vi "COD主界面（列队使用）.vi"() -> (8 "多列列表框":i32(listbox))   [LabVIEW 2016, in "斯坦道CODMn.lvlib"]
uses:
  <vilib>/Plasmionique/MB Master/MB_Master_Serial/MB_Master_Serial.lvclass
  C:/Program Files (x86)/National Instruments/LabVIEW 2016/vi.lib/Plasmionique/MB Master/MB_Master/MB_Master.lvclass
  <vilib>/Analysis/6fits.llb/Curve Fitting Criteria.ctl
  <vilib>/Utility/miscctls.llb/LVPointTypeDef.ctl
  <vilib>/Utility/config.llb/Read Key (Boolean).vi
  <vilib>/Utility/config.llb/Read Key (I32).vi
  <vilib>/Utility/config.llb/Read Key (Double).vi
  <vilib>/Utility/config.llb/Write Key (Double).vi
  <vilib>/Utility/config.llb/Write Key (Boolean).vi
  <vilib>/Utility/config.llb/Write Key (I32).vi
  <vilib>/Plasmionique/MB Master/MB Master.lvlib
  <vilib>/ptbypt/NI_PtbyPt.lvlib
  PLC/PLC.lvlib
  <vilib>/Utility/config.llb/NI_LVConfig.lvlib
  <vilib>/Analysis/NI_AALPro.lvlib
panel:
  out "空白测试标记":bool
  out "跨度核查标记":bool
  out "启动选择 2":u16(ring) items=["水样测试", "标样核查", "零点核查", "跨度核查", "空白测试", "加标回收", "平行样", "校零", "校标"]
  in  "量程选择":enum16{"低量程", "高量程"}(ring)
  out "MB_Serial session":refnum<class "MB_Master_Serial.lvclass">
  in  "手动控制":bool
  in  "选用水样":enum16{"葡萄糖", "草酸钠"}(ring)
  in  "方程系数":cluster{"X^2":dbl, "X":dbl, "b":dbl} {"X^2" format="%#.4g"; "b" format="%#.4g"; "X" format="%#.4g"}
  out "XY图 2":cluster{"X Values":dbl[], "Y Values":dbl[]}[](graph)
  out "多项式系数1":dbl[](array[numeric]) caption="多项式系数"
  out "多项式系数2":dbl[](array[numeric]) caption="多项式系数"
  out "XY图":cluster{"X Values":dbl[], "Y Values":dbl[]}[](graph)
  in  "模型":enum32{"线性", "多项式"}(ring)
  out "启动时间":timestamp format="%<%Y/%m/%d %H:%M:%S>T"
  in  "自动切换量程":bool=TRUE
  in  "24H周期设置":bool[](xcontrol)
  in  "关闭 2":bool
  in  "周期设置":bool
  out "文本.文本":string
  out "r^2":dbl format="%.4g"
  out "r^2":dbl format="%.8g"
  out "高量程拟合方程":string
  out "拟合公式":string
  out "b 2":dbl format="%#.4g"
  out "K 2":dbl format="%#.4g"
  out "b":dbl format="%#.4g"
  out "K":dbl format="%#.4f"
  out "当前校准":i32
  in  "启用3":bool
  in  "启用2":bool
  in  "启用1":bool
  in  "启用6":bool
  in  "启用5":bool
  in  "校准6":bool
  in  "校准5":bool
  in  "校准4":bool
  in  "启用4":bool
  in  "泵滴定数6":dbl
  in  "泵滴定数5":dbl
  in  "泵滴定数4":dbl
  in  "浓度6":dbl
  in  "浓度5":dbl
  in  "浓度4":dbl
  in  "校准3":bool
  in  "校准2":bool
  in  "校准1":bool
  in  "泵滴定数3":dbl
  in  "泵滴定数2":dbl
  in  "泵滴定数1":dbl
  in  "浓度3":dbl
  in  "浓度2":dbl
  in  "浓度1":dbl
  in  "写入":bool
  out "测量模式数字":i32
  out "零点核查标记":bool
  out "排液故障":bool
  out "进水样超量程":bool
  out "标样核查标记":bool
  out "平行样测量":bool
  out "加标回收测量":bool
  out "质控样测量":bool
  out "待机":bool
  out "校标错误":bool
  out "校零错误":bool
  out "测量错误":bool
  out "草酸钠报警":bool
  out "高锰酸钾报警":bool
  out "加热故障":bool
  out "温控器故障":bool
  out "ORP故障":bool
  out "排液标记":bool
  out "故障标记":bool
  out "校标标记":bool
  out "校零标记":bool
  out "通讯状态":bool
  out "水样测量":bool
  out "读取KB值":bool
  in  "读取":bool
  in  "返回":bool
  in  "校准配置":bool
  in  "修正系数 2":dbl
  in  "浓度 2":dbl
  in  "温度":dbl
  in  "恒温时间":dbl
  in  "基本量程":enum16{"10mL", "20mL"}(ring)
  in  "水样":dbl
  in  "蒸馏水":dbl
  in  "标液":dbl
  in  "质控样":dbl
  in  "加标回收":dbl
  in  "草酸钠":dbl
  in  "高锰酸钾":dbl
  in  "硫酸":dbl
  in  "零点泵计量数 2":dbl
  in  "标度泵计量数 2":dbl
  out "标度滴定值":dbl
  out "零点滴定值":dbl
  in  "保存":bool
  in  "关闭":bool
  out "测量数据区":T1 {"单位" items=["ug/L", "mg/L", "ppm", "mg/m3", "cm", "ppb", "ug/m3", "%", "nmol/mol", "umol/mol", "MPN/L", "MPN/100ml", "ng/m3", "NTU", "无量纲", "ms/cm", "us/cm", "℃", "mV", "万个/L"]}
  out "仪器时间":timestamp format="%<%Y/%m/%d %H:%M:%S>T"
  out "秒":u16
  out "分":u16
  out "COD浓度（mg/L)":dbl format="%.2g"
  out "进样管":dbl
  out "高锰酸钾":dbl
  out "草酸钠":dbl
  out "硫酸":dbl
  out "ORP显示":dbl
  out "温度":dbl
  out "加热":bool
  out "搅拌":bool
  out "进硫酸":bool
  out "进加标回收样":bool
  out "进质控样":bool
  out "进标液":bool
  out "进蒸馏水":bool
  out "进水样":bool
  out "进草酸钠":bool
  out "进高锰酸钾":bool
  in  "定时启动":bool
  in  "启动":bool
  in  "故障清除":bool
  in  "参数配置":bool
  in  "停止":bool
  in  "单步启动":bool
  out "定时时间":dbl
  out "系统时间":timestamp
  in  "时间校准":bool
  in  "枚举":enum16{"读取数据", "写入数据", "读取写入DATABASE", "读取参数"}(ring)
  in  "data in":T2
  out "数值":i32
  out "报警簇":T3
  out "读取参数":u16[](array[numeric])
  out "循环次数":i32
  out "DATABASE":u16[](array[numeric])
  out "Registers":u16[](array[numeric])
  in  "Slave ID":u8=1
  in  "Serial Config":T4={"baud rate (bps)"=115200, "stop bits"=10, "parity"=0, "flow control"=0, "timeout"=1000, "retries"=1} {"stop bits" items=["1.0"=10, "1.5"=15, "2.0"=20]; "flow control" items=["None", "XON/XOFF", "RTS/CTS", "XON/XOFF & RTS/CTS", "DTR/DSR", "XON/XOFF & DTR/DSR"]; "parity" items=["None", "Odd", "Even", "Mark", "Space"]}
  out "table 输入":string
  out "columns":string[](array[string])
  out "data":T5
  in  "温度 2":dbl
  in  "浓度":dbl
  in  "修正系数":dbl
  in  "标样浓度 2":dbl
  out "模式（受控）":u16
  in  "VISA resource name":refnum<visa-resource-name>="COM4" caption="VISA资源名称"
  # "测量时间："
  # "水样~加标回收"
  # "mV"
  # "℃"
  # "注：遇到加热故障和排液故障时仪器不能正常启动，\n必须排查故障并点击报警清除按钮方可运行。"
  # "mg/L"
  # "校零校标结果"
  # "基本参数设置"
  # "泵计量参数设置"
  # "校零结果："
  # "校零滴定值："
  # "加热恒温温度（℃）："
  # "水样："
  # "高锰酸钾："
  # "校标结果："
  # "标度滴定值："
  # "零点泵计量值："
  # "恒温时间（分钟）："
  # "蒸馏水："
  # "草酸钠："
  # "标度泵计量值："
  # "标准液浓度（mg/L）："
  # "标液："
  # "标样浓度："
  # "硫酸："
  # "修正系数："
  # "质控样："
  # "基本量程（20mL可选）："
  # "加标回收样："
  # "是否启用"
  # "泵滴定数"
  # "浓度"
  # "辅\n助\n计\n算\n区"
  # "高量程校准"
  # "泵滴定数"
  # "是否启用"
  # "浓度"
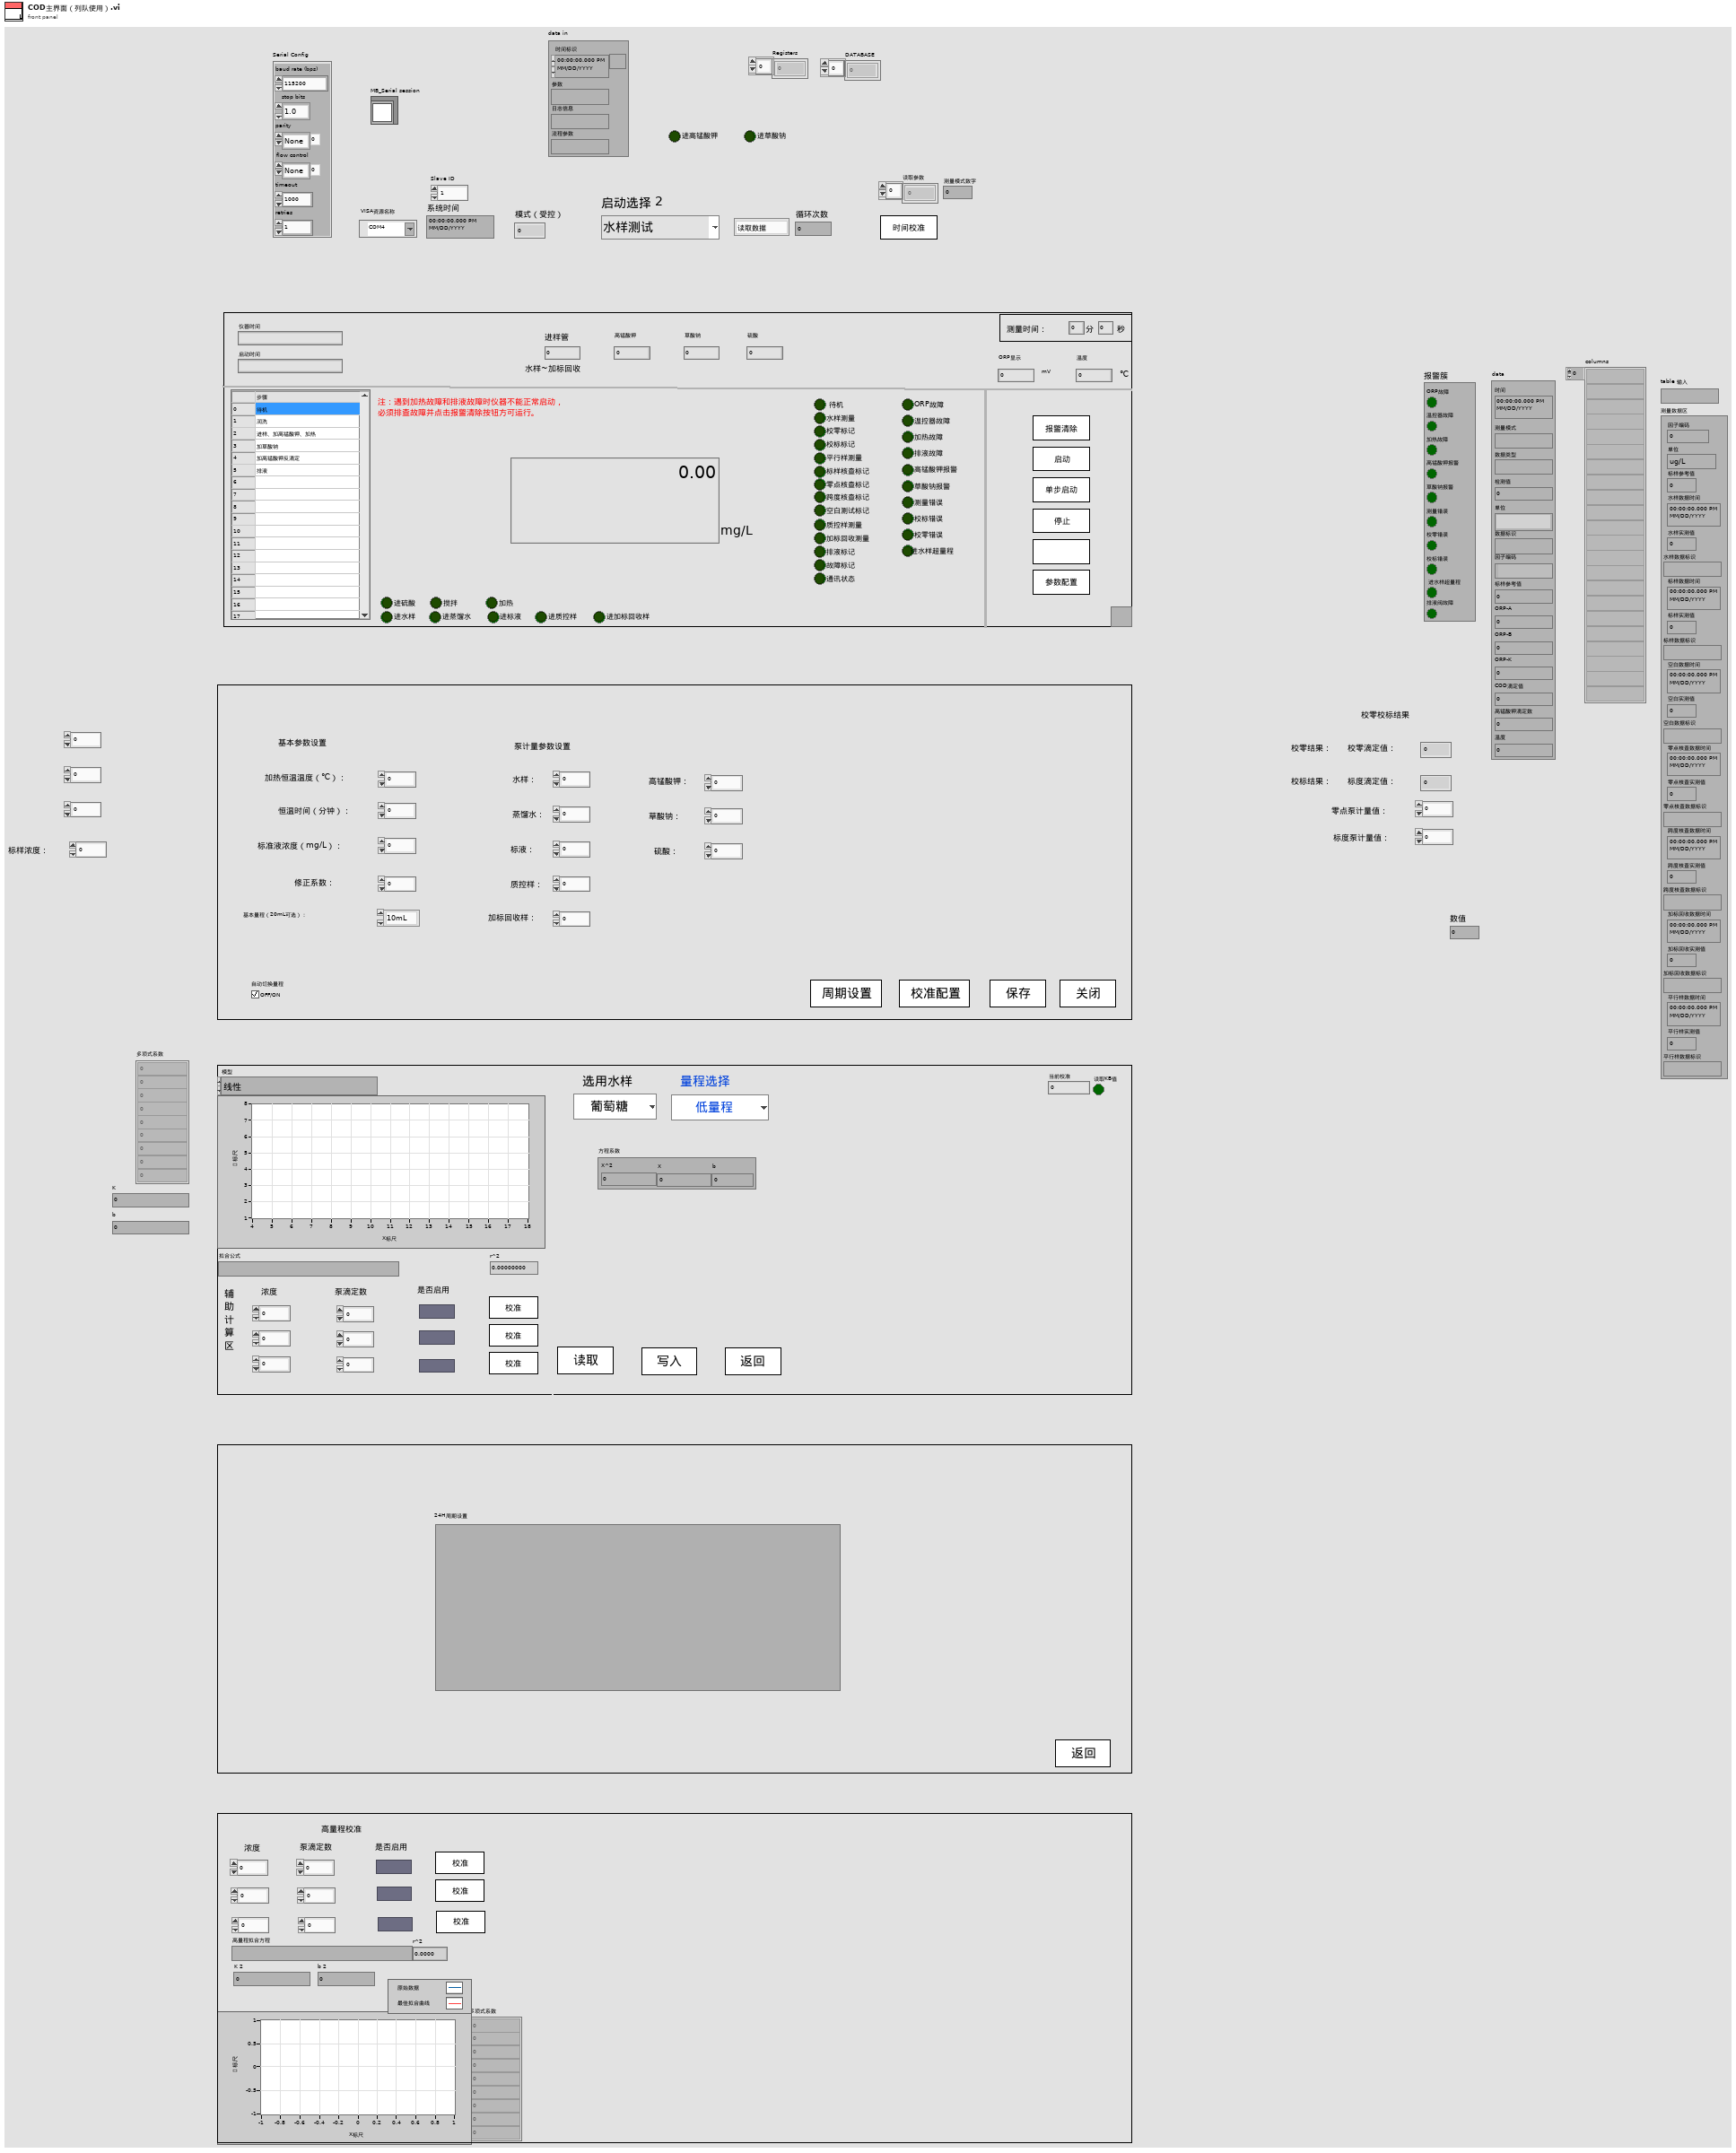
[diagram p1: front panel]
types:
  T1 = cluster{"因子编码":u32, "单位":u16, "标样参考值":sgl, "水样数据时间":timestamp, "水样实测值":sgl, "水样数据标识":string, "标样数据时间":timestamp, "标样实测值":sgl, "标样数据标识":string, "空白数据时间":timestamp, "空白实测值":sgl, "空白数据标识":string, "零点核查数据时间":timestamp, "零点核查实测值":sgl, "零点核查数据标识":string, "跨度核查数据时间":timestamp, "跨度核查实测值":sgl, "跨度核查数据标识":string, "加标回收数据时间":timestamp, "加标回收实测值":sgl, "加标回收数据标识":string, "平行样数据时间":timestamp, "平行样实测值":sgl, "平行样数据标识":string}
  T2 = cluster{"时间标识":timestamp, "参数":string, "日志信息":string, "流程参数":string}
  T3 = cluster{"ORP故障":bool, "温控器故障":bool, "加热故障":bool, "高锰酸钾报警":bool, "草酸钠报警":bool, "测量错误":bool, "校零错误":bool, "校标错误":bool, " 进水样超量程":bool, "排液阀故障":bool}
  T4 = cluster{"baud rate (bps)":u32, "stop bits":u16, "parity":u16, "flow control":u16, "timeout":u32, "retries":i32}
  T5 = cluster{"时间":timestamp, "测量模式":string, "数据类型":string, "检测值":sgl, "单位":string, "数据标识":string, "因子编码":string, "标样参考值":sgl, "ORP-A":sgl, "ORP-B":sgl, "ORP-K":sgl, "COD滴定值":sgl, "高锰酸钾滴定数":sgl, "温度":sgl}
  T6 = cluster{"starting address":u16, "number of holding registers":u16}
  T7 = cluster{"测量模式":enum16{"水样测量", "标样核查", "零点核查", "跨度核查", "空白测试", "加标回收", "平行样", "校零", "校标"}}
  T8 = typedef "LVDateTimeRec.ctl" = cluster{"秒数的小数部分":dbl, "秒":i32, "分":i32, "时":i32, "日":i32, "月":i32, "年":i32, "天数（周）":i32, "天数（年）":i32, "DST":i32}
  T9 = typedef "LVPointTypeDef.ctl" = cluster{"Horizontal":i16, "Vertical":i16}
  T10 = typedef "NI_LVConfig.lvlib/Config Data RefNum.ctl" = refnum<k1>
  T11 = cluster{"时间标识":timestamp, "设备":string, "日志信息":string}
  T12 = typedef "NI_AALPro.lvlib/Curve Fitting Criteria.ctl" = u16
  T13 = cluster{"时间标识":timestamp, "设备":string, "日志信息":string, "流程参数":string}
  T14 = cluster{"数组 2[0]":sgl, "数组 2[1]":sgl, "数组 2[2]":sgl, "数组 2[3]":sgl, "数组 2[4]":sgl, "数组 2[5]":sgl}
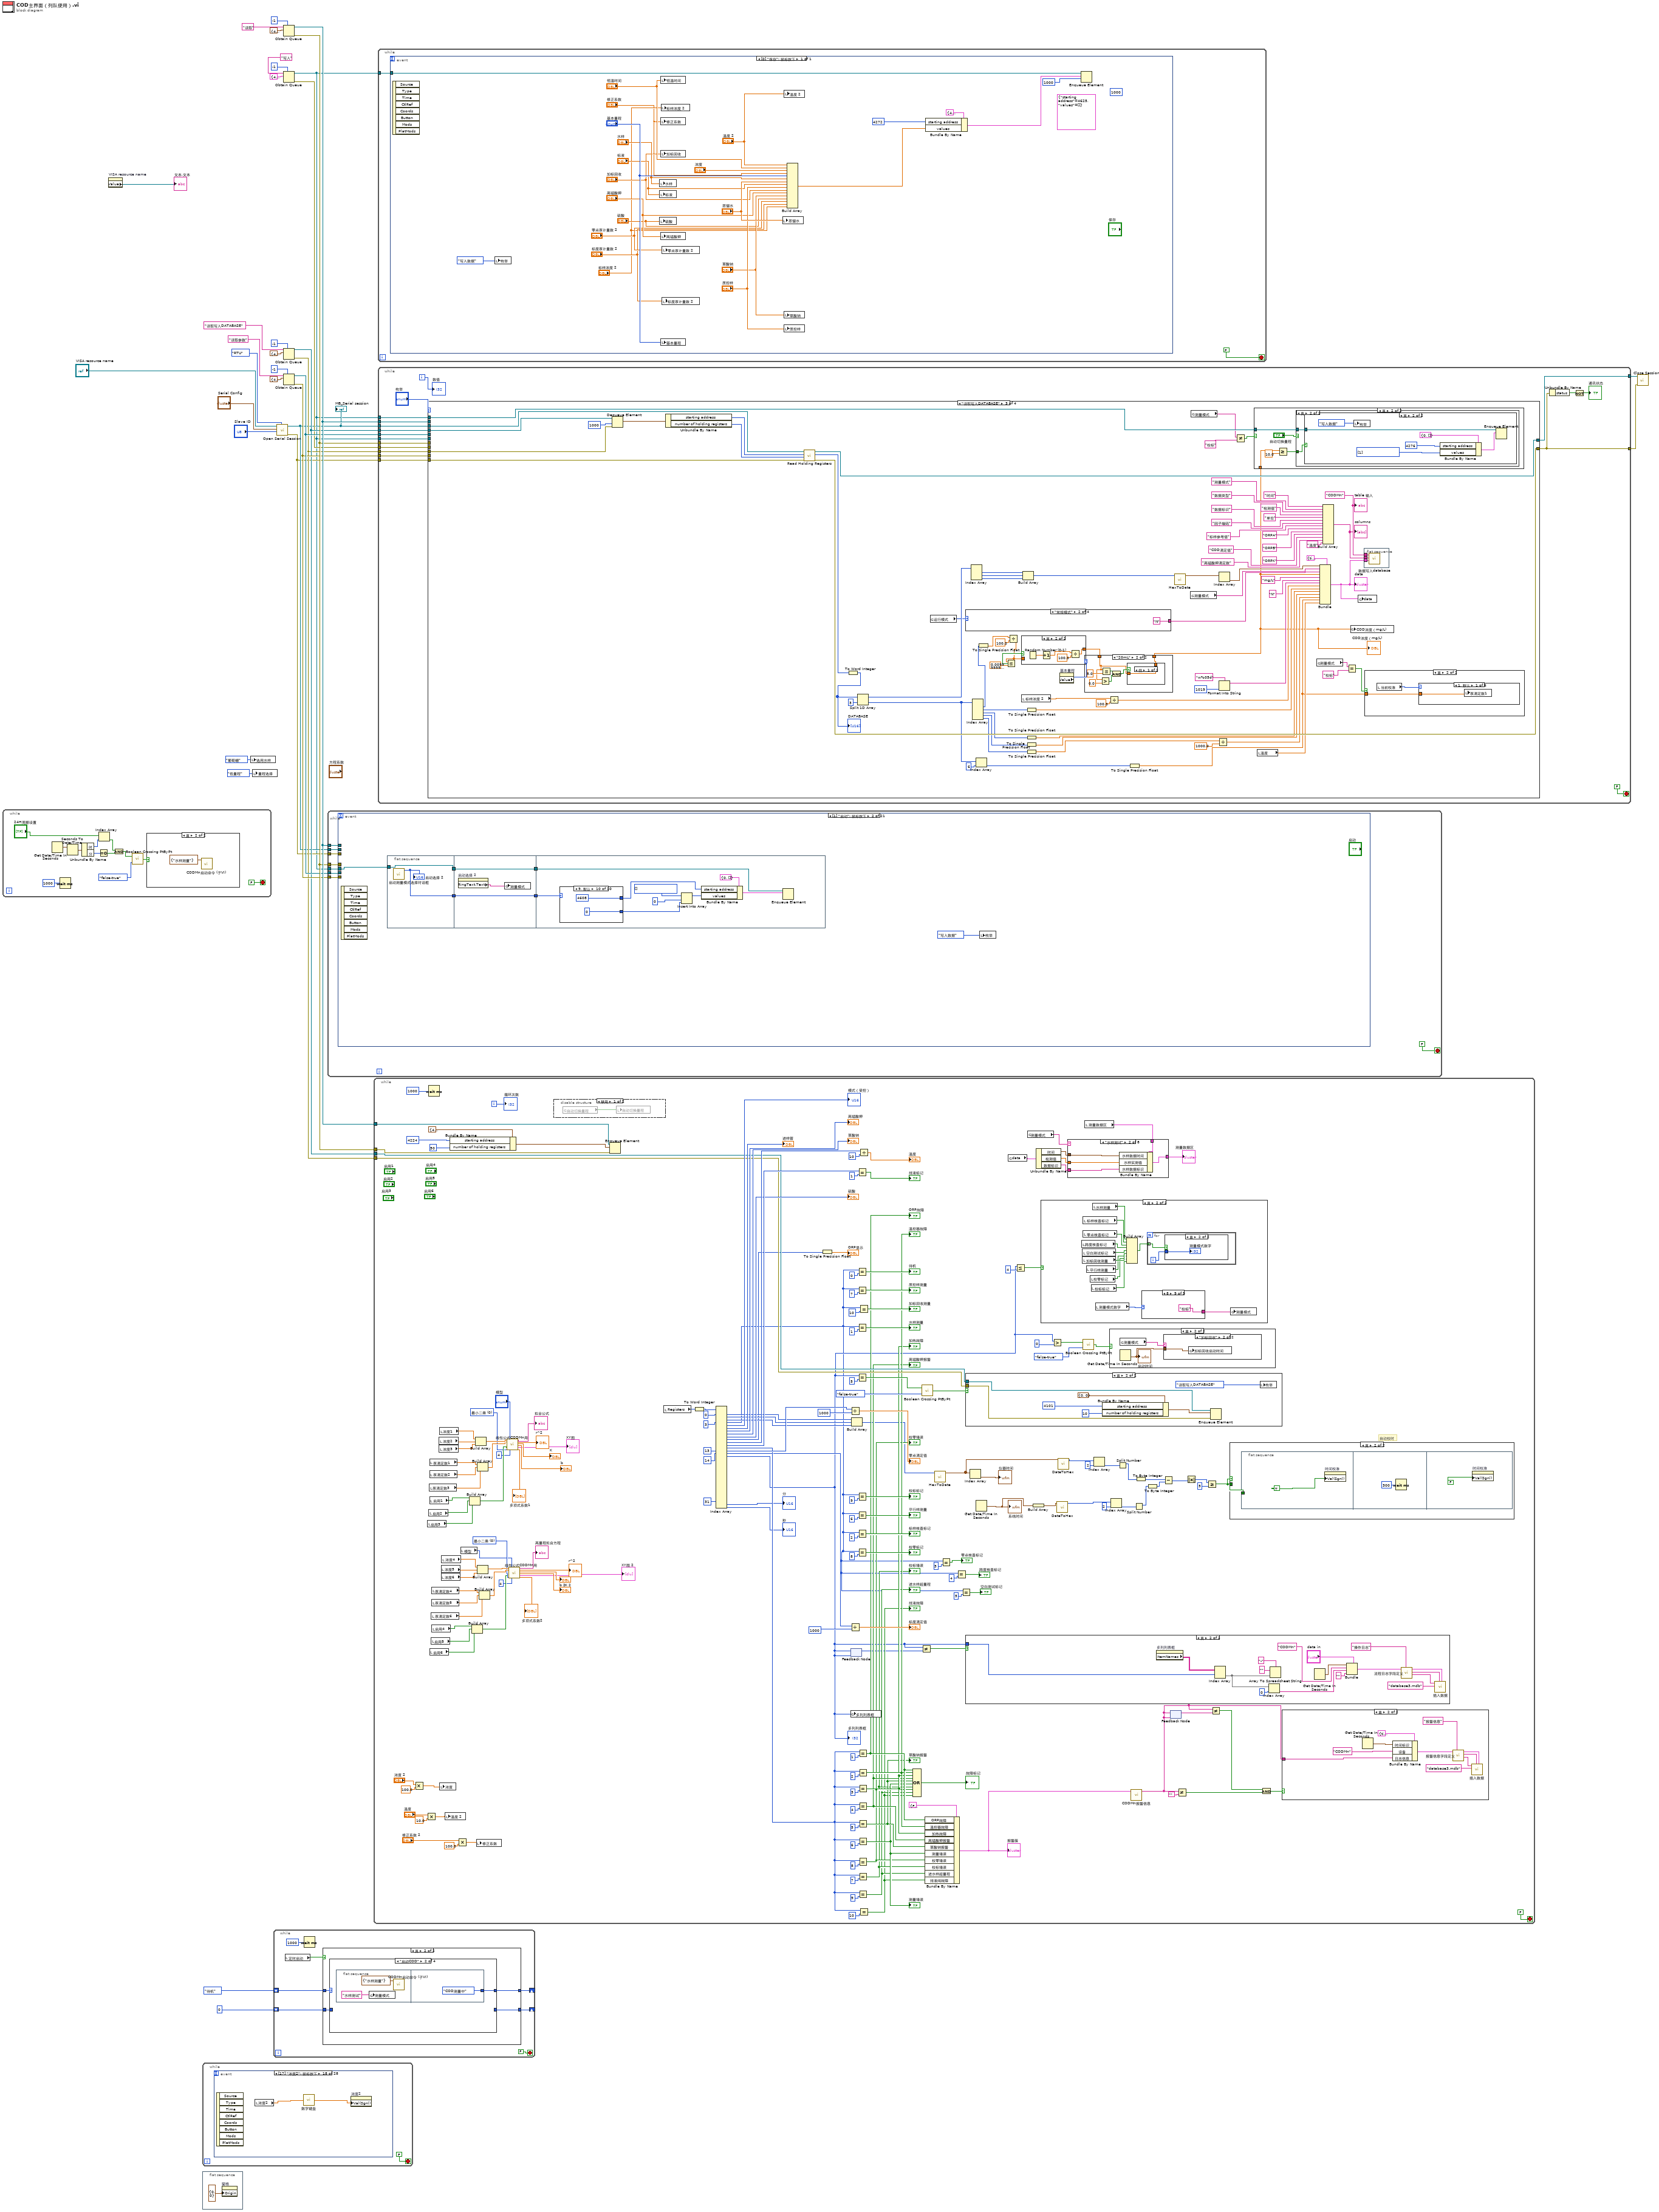
[diagram p0: block diagram]
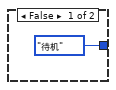
[diagram p3: hidden frame]
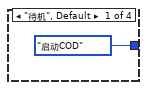
[diagram p4: hidden frame]
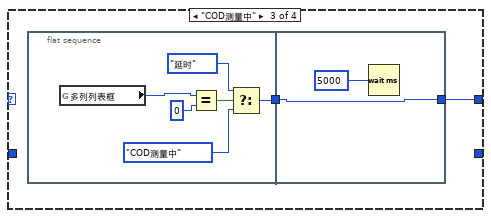
[diagram p5: hidden frame]
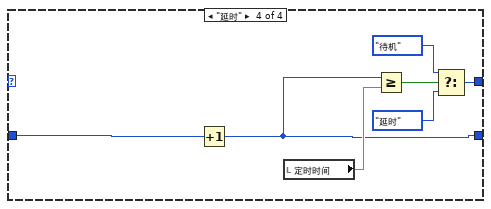
[diagram p6: hidden frame]
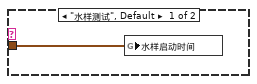
[diagram p9: hidden frame]
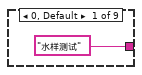
[diagram p11: hidden frame]
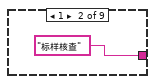
[diagram p12: hidden frame]
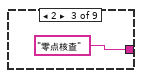
[diagram p13: hidden frame]
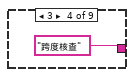
[diagram p14: hidden frame]
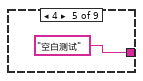
[diagram p15: hidden frame]
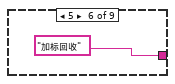
[diagram p16: hidden frame]
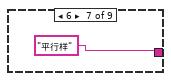
[diagram p17: hidden frame]
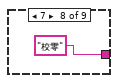
[diagram p18: hidden frame]
diagram:
  n1 = while {
    stop <- FALSE stop-if-true
    n2 = Get Date/Time In Seconds() -> (seconds since 1Jan1904=w45:timestamp)
    n3 = Wait (ms)(milliseconds to wait=u32 1000 ("等待时间（毫秒）")) -> ()  [unwired: 1 out]
    n4 = Seconds To Date/Time(time stamp (now)=w45) -> (date time rec=w44:T8)  [unwired: 1 in]
    n5 = Unbundle By Name(w44) -> ("时"=w41:i32, "分"=w43:i32)
    n6 = Equal To 0?(x=w43) -> (x = 0?=w42:bool)
    n7 = Index Array(array="24H周期设置", index=w41) -> (element=w40:bool)
    n8 = And(x=w40, y=w42) -> (x .and. y?=w38:bool)
    n9 = call <vilib>:"Boolean Crossing PtByPt.vi"("direction"=enum16{"either", "false-true", "true-false"}."false-true", "input"=w38) -> ("crossing"=w37:bool)  [unwired: 1 in]
    n10 = case shown="真" w37 {
      frame False {
      }
      frame True {
        n11 = call "CODMn启动命令 (子VI).vi"("启动测量模式"=T7 {"测量模式"=enum."水样测量"}) -> ()  [unwired: 11 in]
      }
    }
  }
  n12 = property on="VISA resource name" class="VISAName"() -> ("Value"=→"文本.文本":refnum<visa-resource-name>)  [unwired: 2 in, 2 out]
  n13 = while {
    stop <- FALSE stop-if-true
    n14 = event shown="[17] \"浓度2\": 鼠标按下" {
      selector: _ -> [_ _ _ _ _ _ _ _ _ _ _ _ _ _ _ _ _ _ _ _ _ _ _ _ _ _ _ _]
      dyn-events: _ -> [_ _ _ _ _ _ _ _ _ _ _ _ _ _ _ _ _ _ _ _ _ _ _ _ _ _ _ _]
      timeout: _ -> [_ _ _ _ _ _ _ _ _ _ _ _ _ _ _ _ _ _ _ _ _ _ _ _ _ _ _ _]
      event Timeout {
        n15 = event-data() -> ()  [unwired: 1 in, 3 out]
      }
      event "温度": Mouse Down {
        n16 = event-data() -> ()  [unwired: 1 in, 8 out]
        n17 = local read "温度"() -> (w49:dbl)
        n18 = call "数字键盘.vi"("OldNumber"=w49) -> ("NewNumber"=w48:sgl)
        n19 = local write "温度"(w48) -> ()
      }
      event "恒温时间": Mouse Down {
        n20 = event-data() -> ()  [unwired: 1 in, 8 out]
        n21 = local read "恒温时间"() -> (w50:dbl)
        n22 = call "数字键盘.vi"("OldNumber"=w50) -> ("NewNumber"=w51:sgl)
        n23 = local write "恒温时间"(w51) -> ()
      }
      event "浓度 2": Mouse Down {
        n24 = event-data() -> ()  [unwired: 1 in, 8 out]
        n25 = local read "浓度 2"() -> (w53:dbl)
        n26 = call "数字键盘.vi"("OldNumber"=w53) -> ("NewNumber"=w52:sgl)
        n27 = local write "浓度 2"(w52) -> ()
      }
      event "修正系数 2": Mouse Down {
        n28 = event-data() -> ()  [unwired: 1 in, 8 out]
        n29 = local read "修正系数 2"() -> (w54:dbl)
        n30 = call "数字键盘.vi"("OldNumber"=w54) -> ("NewNumber"=w55:sgl)
        n31 = local write "修正系数 2"(w55) -> ()
      }
      event "水样": Mouse Down {
        n32 = event-data() -> ()  [unwired: 1 in, 8 out]
        n33 = local read "水样"() -> (w56:dbl)
        n34 = call "数字键盘.vi"("OldNumber"=w56) -> ("NewNumber"=w57:sgl)
        n35 = local write "水样"(w57) -> ()
      }
      event "蒸馏水": Mouse Down {
        n36 = event-data() -> ()  [unwired: 1 in, 8 out]
        n37 = local read "蒸馏水"() -> (w58:dbl)
        n38 = call "数字键盘.vi"("OldNumber"=w58) -> ("NewNumber"=w59:sgl)
        n39 = local write "蒸馏水"(w59) -> ()
      }
      event "标液": Mouse Down {
        n40 = event-data() -> ()  [unwired: 1 in, 8 out]
        n41 = local read "标液"() -> (w60:dbl)
        n42 = call "数字键盘.vi"("OldNumber"=w60) -> ("NewNumber"=w61:sgl)
        n43 = local write "标液"(w61) -> ()
      }
      event "质控样": Mouse Down {
        n44 = event-data() -> ()  [unwired: 1 in, 8 out]
        n45 = local read "质控样"() -> (w62:dbl)
        n46 = call "数字键盘.vi"("OldNumber"=w62) -> ("NewNumber"=w63:sgl)
        n47 = local write "质控样"(w63) -> ()
      }
      event "加标回收": Mouse Down {
        n48 = event-data() -> ()  [unwired: 1 in, 8 out]
        n49 = local read "加标回收"() -> (w64:dbl)
        n50 = call "数字键盘.vi"("OldNumber"=w64) -> ("NewNumber"=w65:sgl)
        n51 = local write "加标回收"(w65) -> ()
      }
      event "草酸钠": Mouse Down {
        n52 = event-data() -> ()  [unwired: 1 in, 8 out]
        n53 = local read "草酸钠"() -> (w66:dbl)
        n54 = call "数字键盘.vi"("OldNumber"=w66) -> ("NewNumber"=w67:sgl)
        n55 = local write "草酸钠"(w67) -> ()
      }
      event "高锰酸钾": Mouse Down {
        n56 = event-data() -> ()  [unwired: 1 in, 8 out]
        n57 = local read "高锰酸钾"() -> (w68:dbl)
        n58 = call "数字键盘.vi"("OldNumber"=w68) -> ("NewNumber"=w69:sgl)
        n59 = local write "高锰酸钾"(w69) -> ()
      }
      event "硫酸": Mouse Down {
        n60 = event-data() -> ()  [unwired: 1 in, 8 out]
        n61 = local read "硫酸"() -> (w70:dbl)
        n62 = call "数字键盘.vi"("OldNumber"=w70) -> ("NewNumber"=w71:sgl)
        n63 = local write "硫酸"(w71) -> ()
      }
      event "零点泵计量数 2": Mouse Down {
        n64 = event-data() -> ()  [unwired: 1 in, 8 out]
        n65 = local read "零点泵计量数 2"() -> (w72:dbl)
        n66 = call "数字键盘.vi"("OldNumber"=w72) -> ("NewNumber"=w73:sgl)
        n67 = local write "零点泵计量数 2"(w73) -> ()
      }
      event "标度泵计量数 2": Mouse Down {
        n68 = event-data() -> ()  [unwired: 1 in, 8 out]
        n69 = local read "标度泵计量数 2"() -> (w74:dbl)
        n70 = call "数字键盘.vi"("OldNumber"=w74) -> ("NewNumber"=w75:sgl)
        n71 = local write "标度泵计量数 2"(w75) -> ()
      }
      event "标样浓度 2": Mouse Down {
        n72 = event-data() -> ()  [unwired: 1 in, 8 out]
        n73 = local read "标样浓度 2"() -> (w76:dbl)
        n74 = call "数字键盘.vi"("OldNumber"=w76) -> ("NewNumber"=w77:sgl)
        n75 = local write "标样浓度 2"(w77) -> ()
      }
      event "浓度1": Mouse Down {
        n76 = event-data() -> ()  [unwired: 1 in, 8 out]
        n77 = local read "浓度1"() -> (w79:dbl)
        n78 = call "数字键盘.vi"("OldNumber"=w79) -> ("NewNumber"=w78:sgl)
        n79 = property on="浓度1" class="DigNum (严格)"("Val(Sgnl)"=w78) -> ()  [unwired: 2 in, 2 out]
      }
      event "浓度2": Mouse Down {
        n80 = event-data() -> ()  [unwired: 1 in, 8 out]
        n81 = local read "浓度2"() -> (w81:dbl)
        n82 = call "数字键盘.vi"("OldNumber"=w81) -> ("NewNumber"=w80:sgl)
        n83 = property on="浓度2" class="DigNum (严格)"("Val(Sgnl)"=w80) -> ()  [unwired: 2 in, 2 out]
      }
      event "浓度3": Mouse Down {
        n84 = event-data() -> ()  [unwired: 1 in, 8 out]
        n85 = local read "浓度3"() -> (w83:dbl)
        n86 = call "数字键盘.vi"("OldNumber"=w83) -> ("NewNumber"=w82:sgl)
        n87 = property on="浓度3" class="DigNum (严格)"("Val(Sgnl)"=w82) -> ()  [unwired: 2 in, 2 out]
      }
      event "泵滴定数1": Mouse Down {
        n88 = event-data() -> ()  [unwired: 1 in, 8 out]
        n89 = local read "泵滴定数1"() -> (w85:dbl)
        n90 = call "数字键盘.vi"("OldNumber"=w85) -> ("NewNumber"=w84:sgl)
        n91 = property on="泵滴定数1" class="DigNum (严格)"("Val(Sgnl)"=w84) -> ()  [unwired: 2 in, 2 out]
      }
      event "泵滴定数2": Mouse Down {
        n92 = event-data() -> ()  [unwired: 1 in, 8 out]
        n93 = local read "泵滴定数2"() -> (w87:dbl)
        n94 = call "数字键盘.vi"("OldNumber"=w87) -> ("NewNumber"=w86:sgl)
        n95 = property on="泵滴定数2" class="DigNum (严格)"("Val(Sgnl)"=w86) -> ()  [unwired: 2 in, 2 out]
      }
      event "泵滴定数3": Mouse Down {
        n96 = event-data() -> ()  [unwired: 1 in, 8 out]
        n97 = local read "泵滴定数3"() -> (w89:dbl)
        n98 = call "数字键盘.vi"("OldNumber"=w89) -> ("NewNumber"=w88:sgl)
        n99 = property on="泵滴定数3" class="DigNum (严格)"("Val(Sgnl)"=w88) -> ()  [unwired: 2 in, 2 out]
      }
      event "浓度4": Mouse Down {
        n100 = event-data() -> ()  [unwired: 1 in, 8 out]
        n101 = local read "浓度4"() -> (w91:dbl)
        n102 = call "数字键盘.vi"("OldNumber"=w91) -> ("NewNumber"=w90:sgl)
        n103 = property on="浓度4" class="DigNum (严格)"("Val(Sgnl)"=w90) -> ()  [unwired: 2 in, 2 out]
      }
      event "浓度5": Mouse Down {
        n104 = event-data() -> ()  [unwired: 1 in, 8 out]
        n105 = local read "浓度5"() -> (w93:dbl)
        n106 = call "数字键盘.vi"("OldNumber"=w93) -> ("NewNumber"=w92:sgl)
        n107 = property on="浓度5" class="DigNum (严格)"("Val(Sgnl)"=w92) -> ()  [unwired: 2 in, 2 out]
      }
      event "浓度6": Mouse Down {
        n108 = event-data() -> ()  [unwired: 1 in, 8 out]
        n109 = local read "浓度6"() -> (w95:dbl)
        n110 = call "数字键盘.vi"("OldNumber"=w95) -> ("NewNumber"=w94:sgl)
        n111 = property on="浓度6" class="DigNum (严格)"("Val(Sgnl)"=w94) -> ()  [unwired: 2 in, 2 out]
      }
      event "泵滴定数4": Mouse Down {
        n112 = event-data() -> ()  [unwired: 1 in, 8 out]
        n113 = local read "泵滴定数4"() -> (w97:dbl)
        n114 = call "数字键盘.vi"("OldNumber"=w97) -> ("NewNumber"=w96:sgl)
        n115 = property on="泵滴定数4" class="DigNum (严格)"("Val(Sgnl)"=w96) -> ()  [unwired: 2 in, 2 out]
      }
      event "泵滴定数5": Mouse Down {
        n116 = event-data() -> ()  [unwired: 1 in, 8 out]
        n117 = local read "泵滴定数5"() -> (w99:dbl)
        n118 = call "数字键盘.vi"("OldNumber"=w99) -> ("NewNumber"=w98:sgl)
        n119 = property on="泵滴定数5" class="DigNum (严格)"("Val(Sgnl)"=w98) -> ()  [unwired: 2 in, 2 out]
      }
      event "泵滴定数6": Mouse Down {
        n120 = event-data() -> ()  [unwired: 1 in, 8 out]
        n121 = local read "泵滴定数6"() -> (w101:dbl)
        n122 = call "数字键盘.vi"("OldNumber"=w101) -> ("NewNumber"=w100:sgl)
        n123 = property on="泵滴定数6" class="DigNum (严格)"("Val(Sgnl)"=w100) -> ()  [unwired: 2 in, 2 out]
      }
    }
  }
  n124 = flat-sequence {
    frame #0 {
      n125 = property on="窗格" class="Pane"("Origin"=T9 {"Horizontal"=0, "Vertical"=0} ("原点")) -> ()  [unwired: 2 in, 2 out]
    }
  }
  n126 = local write "选用水样"(enum16{"葡萄糖", "草酸钠"}."葡萄糖" ("选用水样")) -> ()
  n127 = local write "量程选择"(enum16{"低量程", "高量程"}."低量程" ("量程选择")) -> ()
  n128 = while {
    shift-right: [w104] -> _
    shift-left: enum16{"待机", "启动COD", "COD测量中", "延时"}."待机" -> [w106]
    shift-right: [w103] -> _
    shift-left: 0 -> [w105]
    stop <- FALSE stop-if-true
    n129 = local read "定时启动"() -> (w108:bool)
    n130 = Wait (ms)(milliseconds to wait=u32 1000 ("等待时间（毫秒）")) -> ()  [unwired: 1 out]
    n131 = case shown="真" w108 {
      tunnel: w106 -> [_ w114]
      tunnel: w105 -> [_ w113]
      tunnel: [enum16{"待机", "启动COD", "COD测量中", "延时"}."待机" w112] -> w104
      tunnel: [_ w111] -> w103
      frame False {
      }
      frame True {
        n132 = case shown="\"启动COD\"" w114 {
          tunnel: w113 -> [_ _ _ w136]
          tunnel: [enum16{"待机", "启动COD", "COD测量中", "延时"}."启动COD" w116 w121 w130] -> w112
          tunnel: [_ _ _ w133] -> w111
          frame "待机", Default {
          }
          frame "启动COD" {
            n133 = flat-sequence {
              tunnel: [enum16{"待机", "启动COD", "COD测量中", "延时"}."COD测量中"] -> w116
              frame #0 {
                n134 = global write "COD测量模式全局.vi" "测量模式"("水样测试" ("测量模式")) -> ()
                n135 = call "CODMn启动命令 (子VI).vi"("启动测量模式"=T7 {"测量模式"=enum."水样测量"}) -> ()  [unwired: 11 in]
              }
              frame #1 {
              }
            }
          }
          frame "COD测量中" {
            n136 = flat-sequence {
              tunnel: [w122] -> w120
              tunnel: [w129] -> w121
              tunnel: w120 -> [w129]
              frame #0 {
                n137 = global read "运行时序全局变量.vi" "多列列表框"() -> (w127:i32)
                n138 = Equal?(x=w127, y=0) -> (x = y?=w125:bool)
                n139 = Select(t=enum16{"待机", "启动COD", "COD测量中", "延时"}."延时", s=w125, f=enum16{"待机", "启动COD", "COD测量中", "延时"}."COD测量中") -> (s? t:f=w122:enum16{"待机", "启动COD", "COD测量中", "延时"})
              }
              frame #1 {
                n140 = Wait (ms)(milliseconds to wait=u32 5000 ("等待时间（毫秒）")) -> ()  [unwired: 1 out]
              }
            }
          }
          frame "延时" {
            n141 = Increment(x=w136) -> (x+1=w133:i32)
            n142 = local read "定时时间"() -> (w135:dbl)
            n143 = Greater Or Equal?(x=w133, y=w135) -> (x >= y?=w134:bool)
            n144 = Select(t=enum16{"待机", "启动COD", "COD测量中", "延时"}."待机", s=w134, f=enum16{"待机", "启动COD", "COD测量中", "延时"}."延时") -> (s? t:f=w130:enum16{"待机", "启动COD", "COD测量中", "延时"})
          }
        }
      }
    }
  }
  n145 = call <vilib>:"Open Serial Session.vi"("Mode (RTU)"=enum16{"RTU", "ASCII"}."RTU", "Slave ID"="Slave ID", "Serial Config"="Serial Config", "VISA Resource"="VISA resource name") -> ("Error out"=w7:errorcluster, "MB_Serial session"=w8:refnum<class "MB_Master_Serial.lvclass">)  [unwired: 6 in]
  "MB_Serial session" <- w8
  n146 = Obtain Queue(max queue size (-1, unlimited)=-1 ("队列最大值（-1，无限）"), name (unnamed)="读取" ("名称（未命名）"), element data type=T6 {"starting address"=4224, "number of holding registers"=16}) -> (queue out=w23:refnum<queue>, error out=w22:errorcluster)  [unwired: 2 in, 1 out]
  n147 = Obtain Queue(max queue size (-1, unlimited)=-1 ("队列最大值（-1，无限）"), name (unnamed)="写入" ("名称（未命名）"), element data type=cluster{"starting address":u16, "values":u16[]} {"starting address"=4272, "values"=[]}) -> (queue out=w4:refnum<queue>, error out=w9:errorcluster)  [unwired: 2 in, 1 out]
  n148 = Obtain Queue(max queue size (-1, unlimited)=-1 ("队列最大值（-1，无限）"), name (unnamed)="读取写入DATABASE" ("名称（未命名）"), element data type=T6 {"starting address"=4224, "number of holding registers"=16}) -> (queue out=w11:refnum<queue>, error out=w10:errorcluster)  [unwired: 2 in, 1 out]
  n149 = Obtain Queue(max queue size (-1, unlimited)=-1 ("队列最大值（-1，无限）"), name (unnamed)="读取参数" ("名称（未命名）"), element data type=T6 {"starting address"=4224, "number of holding registers"=16}) -> (queue out=w16:refnum<queue>, error out=w15:errorcluster)  [unwired: 2 in, 1 out]
  n150 = while {
    tunnel: w23 -> [w144]
    tunnel: w22 -> [w143]
    tunnel: w4 -> [w142]
    tunnel: w16 -> [w141]
    tunnel: w15 -> [w140]
    tunnel: w8 -> [w138]
    tunnel: w7 -> [w137]
    stop <- FALSE stop-if-true
    n151 = event shown="[1] \"启动\": 鼠标按下" {
      selector: _ -> [_ _ _ _ _ _ _ _ _ _ _ _ _ _ _ _ _ _ _ _ _]
      dyn-events: _ -> [_ _ _ _ _ _ _ _ _ _ _ _ _ _ _ _ _ _ _ _ _]
      timeout: _ -> [_ _ _ _ _ _ _ _ _ _ _ _ _ _ _ _ _ _ _ _ _]
      tunnel: w144 -> [_ _ _ _ _ _ _ _ _ _ _ _ _ _ _ _ _ _ _ _ _]
      tunnel: w143 -> [_ _ _ _ _ _ _ _ _ _ _ _ _ _ _ _ _ _ _ _ _]
      tunnel: w142 -> [w152 w185 w222 _ _ _ _ _ _ _ _ _ w623 w637 _ w645 _ _ _ _ w838]
      tunnel: w141 -> [_ _ _ _ w241 _ _ _ _ _ _ _ _ _ _ _ _ _ _ w830 _]
      tunnel: w140 -> [_ _ _ _ w240 _ _ _ _ _ _ _ _ _ _ _ _ _ _ w829 _]
      tunnel: w138 -> [_ _ _ w228 _ _ _ _ _ _ _ w622 _ _ _ _ _ _ _ _ _]
      tunnel: w137 -> [_ _ _ w227 _ _ _ _ _ _ _ w621 _ _ _ _ _ _ _ _ _]
      event "单步启动": Mouse Down {
        n152 = event-data() -> ()  [unwired: 1 in, 8 out]
        n153 = call "单步启动选择对话框.vi"() -> ("启动选择2"=w145:u16)  [unwired: 10 in, 1 out]
        n154 = case shown="12, 默认" w145 {
          tunnel: [u16 4610 ("address") u16 4610 ("address") u16 4610 ("address") u16 4610 ("address") u16 4610 ("address") u16 4610 ("address") u16 4610 ("address") u16 4610 ("address") u16 4610 ("address") u16 4610 ("address") u16 4610 ("address") u16 4610 ("address") u16 4610 ("address")] -> w151
          tunnel: [u16 1 ("address") u16 2 ("address") u16 3 ("address") u16 4 ("address") u16 5 ("address") u16 6 ("address") u16 7 ("address") u16 8 ("address") u16 9 ("holding register value") u16 10 ("holding register value") u16 11 ("holding register value") u16 12 ("address") u16 0 ("address")] -> w148
          frame 0 {
          }
          frame 1 {
          }
          frame 2 {
          }
          frame 3 {
          }
          frame 4 {
          }
          frame 5 {
          }
          frame 6 {
          }
          frame 7 {
          }
          frame 8 {
          }
          frame 9 {
          }
          frame 10 {
          }
          frame 11 {
          }
          frame 12, Default {
          }
        }
        n155 = local write "枚举"(enum16{"读取数据", "写入数据", "读取写入DATABASE", "读取参数"}."写入数据" ("枚举")) -> ()
        n156 = Insert Into Array(array=u16[] [] ("values"), index=0 ("索引"), new element=w148) -> (w147:u16[])
        n157 = Bundle By Name(cluster=cluster{"starting address":u16, "values":u16[]} {"starting address"=0, "values"=[]}, "starting address"=w151, "values"=w147) -> (w153:cluster{"starting address":u16, "values":u16[]})
        n158 = Enqueue Element(queue=w152, element=w153) -> ()  [unwired: 2 in, 3 out]
      }
      event "启动": Mouse Down {
        n159 = event-data() -> ()  [unwired: 1 in, 8 out]
        n160 = flat-sequence {
          tunnel: w185 -> [w188]
          tunnel: [w188] -> w184
          tunnel: [w187] -> w181
          tunnel: w184 -> [w191]
          tunnel: [w191] -> w183
          tunnel: [w189] -> w182
          tunnel: w181 -> [w189]
          tunnel: w183 -> [w193]
          tunnel: w182 -> [w192]
          frame #0 {
            n161 = call "启动测量模式选择对话框.vi"() -> ("启动选择 2"=w187:u16)  [unwired: 11 in]
            "启动选择 2" <- w187
          }
          frame #1 {
            n162 = property on="启动选择 2" class="Ring (严格)"() -> ("RingText.Text"=w190:string)  [unwired: 2 in, 2 out]
            n163 = global write "COD测量模式全局.vi" "测量模式"(w190) -> ()
          }
          frame #2 {
            n164 = case shown="9, 默认" w192 {
              tunnel: [u16 4608 ("address") u16 4608 ("address") u16 4608 ("address") u16 4608 ("address") u16 4608 ("address") u16 4608 ("address") u16 4608 ("address") u16 4608 ("address") u16 4608 ("address") u16 4608 ("address")] -> w194
              tunnel: [u16 1 ("address") u16 2 ("address") u16 3 ("address") u16 4 ("address") u16 5 ("address") u16 7 ("address") u16 6 ("address") u16 8 ("address") u16 9 ("address") u16 0 ("address")] -> w195
              frame 0 {
              }
              frame 1 {
              }
              frame 2 {
              }
              frame 3 {
              }
              frame 4 {
              }
              frame 5 {
              }
              frame 6 {
              }
              frame 7 {
              }
              frame 8 {
              }
              frame 9, Default {
              }
            }
            n165 = Insert Into Array(array=u16[] [] ("values"), index=0 ("索引"), new element=w195) -> (w200:u16[])
            n166 = Bundle By Name(cluster=cluster{"starting address":u16, "values":u16[]} {"starting address"=0, "values"=[]}, "starting address"=w194, "values"=w200) -> (w197:cluster{"starting address":u16, "values":u16[]})
            n167 = Enqueue Element(queue=w193, element=w197) -> ()  [unwired: 2 in, 3 out]
          }
        }
        n168 = local write "枚举"(enum16{"读取数据", "写入数据", "读取写入DATABASE", "读取参数"}."写入数据" ("枚举")) -> ()
      }
      event "停止": Value Change {
        n169 = event-data() -> ()  [unwired: 1 in, 6 out]
        n170 = local write "枚举"(enum16{"读取数据", "写入数据", "读取写入DATABASE", "读取参数"}."写入数据" ("枚举")) -> ()
        n171 = Bundle By Name(cluster=cluster{"starting address":u16, "values":u16[]} {"starting address"=0, "values"=[]}, "starting address"=u16 4608, "values"=u16[] [11]) -> (w224:cluster{"starting address":u16, "values":u16[]})
        n172 = Enqueue Element(queue=w222, element=w224) -> ()  [unwired: 2 in, 3 out]
      }
      event "手动控制": Value Change {
        n173 = event-data() -> ()  [unwired: 1 in, 6 out]
        n174 = call "CODMn手动控制框.vi"("Error in"=w227, "MB_Serial session"=w228) -> ()  [unwired: 10 in]
      }
      event "参数配置": Value Change {
        n175 = event-data() -> ()  [unwired: 1 in, 6 out]
        n176 = property on="窗格" class="Pane"("Origin"=T9 {"Horizontal"=0, "Vertical"=650} ("原点")) -> ()  [unwired: 2 in, 2 out]
        n177 = Bundle By Name(cluster=T6 {"starting address"=0, "number of holding registers"=0}, "starting address"=u16 4240, "number of holding registers"=u16 16) -> (w248:T6)
        n178 = local write "读取KB值"(FALSE ("读取KB值")) -> ()
        n179 = local write "枚举"(enum16{"读取数据", "写入数据", "读取写入DATABASE", "读取参数"}."读取参数" ("枚举")) -> ()
        n180 = Flush Queue(queue=w241, error in (no error)=w240) -> (queue out=w244:refnum<queue>, error out=w243:errorcluster)  [unwired: 1 out]
        n181 = Enqueue Element(queue=w244, element=w248, error in (no error)=w243) -> ()  [unwired: 1 in, 3 out]
        n182 = call <vilib>:"Application Directory.vi"() -> ("Application Directory"=w236:path)
        n183 = Build Path(base path=w236, name or relative path="data\\Set.ini" ("名称或相对路径")) -> (appended path=w234:path)
        n184 = call <vilib>:"Open Config Data.vi"("configuration file path"=w234) -> ("error out"=w237:errorcluster, "refnum"=w238:T10)  [unwired: 8 in, 1 out]
        n185 = call-poly <vilib>:"Read Key.vi"("section"="CODMn是否切换量程" ("key"), "error in (no error)"=w237, "key"="自动切换量程", "refnum"=w238) -> ("error out"=w230:errorcluster, "value"=w229:bool, "refnum out"=w231:T10)  [unwired: 4 in, 1 out]
        n186 = local write "自动切换量程"(w229) -> ()
        n187 = call <vilib>:"Close Config Data.vi"("error in (no error)"=w230, "refnum"=w231) -> ()  [unwired: 8 in, 2 out]
      }
      event "校准配置": Value Change {
        n188 = event-data() -> ()  [unwired: 1 in, 6 out]
        n189 = property on="窗格" class="Pane"("Origin"=T9 {"Horizontal"=0, "Vertical"=1300} ("原点")) -> ()  [unwired: 2 in, 2 out]
        n190 = call <vilib>:"Application Directory.vi"() -> ("Application Directory"=w298:path)
        n191 = Build Path(base path=w298, name or relative path="data\\Set.ini" ("名称或相对路径")) -> (appended path=w296:path)
        n192 = call <vilib>:"Open Config Data.vi"("configuration file path"=w296) -> ("error out"=w258:errorcluster, "refnum"=w259:T10)  [unwired: 8 in, 1 out]
        n193 = call-poly <vilib>:"Read Key.vi"("section"="CODMn模型选择" ("key"), "error in (no error)"=w258, "key"="线性和多项式", "refnum"=w259) -> ("error out"=w254:errorcluster, "value"=w257:i32, "refnum out"=w255:T10)  [unwired: 4 in, 1 out]
        n194 = local write "模型"(w257) -> ()
        n195 = call-poly <vilib>:"Read Key.vi"("section"="标线选择", "error in (no error)"=w254, "key"="选用水样", "refnum"=w255) -> ("error out"=w252:errorcluster, "value"=w256:i32, "refnum out"=w253:T10)  [unwired: 4 in, 1 out]
        n196 = local write "选用水样"(w256) -> ()
        n197 = local read "量程选择"() -> (w265:enum16{"低量程", "高量程"})
        n198 = case shown="0, 默认" w256 {
          tunnel: ["葡萄糖标线" ("section") "草酸钠标线" ("section")] -> w264
          frame 0, Default {
          }
          frame 1 {
          }
        }
        n199 = case shown="\"高量程\"" w265 {
          tunnel: ["低量程" "高量程"] -> w263
          frame "低量程", Default {
          }
          frame "高量程" {
          }
        }
        n200 = Concatenate Strings(w264, w263) -> (w262:string)
        n201 = call-poly <vilib>:"Read Key.vi"("section"=w262, "error in (no error)"=w252, "key"="浓度1", "refnum"=w253) -> ("error out"=w302:errorcluster, "value"=w300:dbl, "refnum out"=w301:T10)  [unwired: 4 in, 1 out]
        n202 = local write "浓度1"(w300) -> ()
        n203 = call-poly <vilib>:"Read Key.vi"("section"=w262, "error in (no error)"=w302, "key"="浓度2", "refnum"=w301) -> ("error out"=w316:errorcluster, "value"=w303:dbl, "refnum out"=w315:T10)  [unwired: 4 in, 1 out]
        n204 = local write "浓度2"(w303) -> ()
        n205 = call-poly <vilib>:"Read Key.vi"("section"=w262, "error in (no error)"=w316, "key"="浓度3", "refnum"=w315) -> ("error out"=w317:errorcluster, "value"=w305:dbl, "refnum out"=w314:T10)  [unwired: 4 in, 1 out]
        n206 = local write "浓度3"(w305) -> ()
        n207 = call-poly <vilib>:"Read Key.vi"("section"=w262, "error in (no error)"=w317, "key"="泵滴定数1", "refnum"=w314) -> ("error out"=w318:errorcluster, "value"=w307:dbl, "refnum out"=w313:T10)  [unwired: 4 in, 1 out]
        n208 = local write "泵滴定数1"(w307) -> ()
        n209 = call-poly <vilib>:"Read Key.vi"("section"=w262, "error in (no error)"=w318, "key"="泵滴定数2", "refnum"=w313) -> ("error out"=w312:errorcluster, "value"=w310:dbl, "refnum out"=w319:T10)  [unwired: 4 in, 1 out]
        n210 = local write "泵滴定数2"(w310) -> ()
        n211 = call-poly <vilib>:"Read Key.vi"("section"=w262, "error in (no error)"=w312, "key"="泵滴定数3", "refnum"=w319) -> ("error out"=w327:errorcluster, "value"=w326:dbl, "refnum out"=w320:T10)  [unwired: 4 in, 1 out]
        n212 = local write "泵滴定数3"(w326) -> ()
        n213 = call-poly <vilib>:"Read Key.vi"("section"=w262, "error in (no error)"=w327, "key"="浓度4", "refnum"=w320) -> ("error out"=w328:errorcluster, "value"=w334:dbl, "refnum out"=w321:T10)  [unwired: 4 in, 1 out]
        n214 = local write "浓度4"(w334) -> ()
        n215 = call-poly <vilib>:"Read Key.vi"("section"=w262, "error in (no error)"=w328, "key"="浓度5", "refnum"=w321) -> ("error out"=w329:errorcluster, "value"=w335:dbl, "refnum out"=w322:T10)  [unwired: 4 in, 1 out]
        n216 = local write "浓度5"(w335) -> ()
        n217 = call-poly <vilib>:"Read Key.vi"("section"=w262, "error in (no error)"=w329, "key"="浓度6", "refnum"=w322) -> ("error out"=w330:errorcluster, "value"=w336:dbl, "refnum out"=w323:T10)  [unwired: 4 in, 1 out]
        n218 = local write "浓度6"(w336) -> ()
        n219 = call-poly <vilib>:"Read Key.vi"("section"=w262, "error in (no error)"=w330, "key"="泵滴定数4", "refnum"=w323) -> ("error out"=w331:errorcluster, "value"=w337:dbl, "refnum out"=w324:T10)  [unwired: 4 in, 1 out]
        n220 = local write "泵滴定数4"(w337) -> ()
        n221 = call-poly <vilib>:"Read Key.vi"("section"=w262, "error in (no error)"=w331, "key"="泵滴定数5", "refnum"=w324) -> ("error out"=w332:errorcluster, "value"=w338:dbl, "refnum out"=w325:T10)  [unwired: 4 in, 1 out]
        n222 = local write "泵滴定数5"(w338) -> ()
        n223 = call-poly <vilib>:"Read Key.vi"("section"=w262, "error in (no error)"=w332, "key"="泵滴定数6", "refnum"=w325) -> ("error out"=w292:errorcluster, "value"=w339:dbl, "refnum out"=w295:T10)  [unwired: 4 in, 1 out]
        n224 = local write "泵滴定数6"(w339) -> ()
        n225 = call-poly <vilib>:"Read Key.vi"("section"=w262, "error in (no error)"=w292, "key"="当前选用的校准", "refnum"=w295) -> ("error out"=w290:errorcluster, "value"=w293:i32, "refnum out"=w291:T10)  [unwired: 4 in, 1 out]
        n226 = local write "当前校准"(w293) -> ()
        n227 = call-poly <vilib>:"Read Key.vi"("section"=w262, "error in (no error)"=w290, "key"="启用1", "refnum"=w291) -> ("error out"=w287:errorcluster, "value"=w273:bool, "refnum out"=w288:T10)  [unwired: 4 in, 1 out]
        n228 = local write "启用1"(w273) -> ()
        n229 = call-poly <vilib>:"Read Key.vi"("section"=w262, "error in (no error)"=w287, "key"="启用2", "refnum"=w288) -> ("error out"=w285:errorcluster, "value"=w272:bool, "refnum out"=w286:T10)  [unwired: 4 in, 1 out]
        n230 = local write "启用2"(w272) -> ()
        n231 = call-poly <vilib>:"Read Key.vi"("section"=w262, "error in (no error)"=w285, "key"="启用3", "refnum"=w286) -> ("error out"=w283:errorcluster, "value"=w271:bool, "refnum out"=w284:T10)  [unwired: 4 in, 1 out]
        n232 = local write "启用3"(w271) -> ()
        n233 = call-poly <vilib>:"Read Key.vi"("section"=w262, "error in (no error)"=w283, "key"="启用4", "refnum"=w284) -> ("error out"=w281:errorcluster, "value"=w270:bool, "refnum out"=w282:T10)  [unwired: 4 in, 1 out]
        n234 = local write "启用4"(w270) -> ()
        n235 = call-poly <vilib>:"Read Key.vi"("section"=w262, "error in (no error)"=w281, "key"="启用5", "refnum"=w282) -> ("error out"=w279:errorcluster, "value"=w269:bool, "refnum out"=w280:T10)  [unwired: 4 in, 1 out]
        n236 = local write "启用5"(w269) -> ()
        n237 = call-poly <vilib>:"Read Key.vi"("section"=w262, "error in (no error)"=w279, "key"="启用6", "refnum"=w280) -> ("error out"=w250:errorcluster, "value"=w268:bool, "refnum out"=w251:T10)  [unwired: 4 in, 1 out]
        n238 = local write "启用6"(w268) -> ()
        n239 = call <vilib>:"Close Config Data.vi"("error in (no error)"=w250, "refnum"=w251) -> ()  [unwired: 8 in, 2 out]
      }
      event "选用水样": Value Change {
        (unwired) "选用水样" ("key")
        (unwired) "标线选择" ("section")
        n240 = event-data() -> ()  [unwired: 1 in, 6 out]
        n241 = property on="窗格" class="Pane"("Origin"=T9 {"Horizontal"=0, "Vertical"=1300} ("原点")) -> ()  [unwired: 2 in, 2 out]
        n242 = local read "量程选择"() -> (w351:enum16{"低量程", "高量程"})
        n243 = case shown="\"高量程\"" w351 {
          tunnel: ["低量程" "高量程"] -> w352
          frame "低量程", Default {
          }
          frame "高量程" {
          }
        }
        n244 = case shown="\"葡萄糖\", 默认" "选用水样" {
          tunnel: ["葡萄糖标线" ("section") "草酸钠标线" ("section")] -> w353
          frame "葡萄糖", Default {
          }
          frame "草酸钠" {
          }
        }
        n245 = call <vilib>:"Application Directory.vi"() -> ("Application Directory"=w387:path)
        n246 = Build Path(base path=w387, name or relative path="data\\Set.ini" ("名称或相对路径")) -> (appended path=w385:path)
        n247 = call <vilib>:"Open Config Data.vi"("configuration file path"=w385) -> ("error out"=w388:errorcluster, "refnum"=w389:T10)  [unwired: 8 in, 1 out]
        n248 = Concatenate Strings(w353, w352) -> (w350:string)
        n249 = call-poly <vilib>:"Read Key.vi"("section"=w350, "error in (no error)"=w388, "key"="浓度1", "refnum"=w389) -> ("error out"=w393:errorcluster, "value"=w391:dbl, "refnum out"=w392:T10)  [unwired: 4 in, 1 out]
        n250 = local write "浓度1"(w391) -> ()
        n251 = call-poly <vilib>:"Read Key.vi"("section"=w350, "error in (no error)"=w393, "key"="浓度2", "refnum"=w392) -> ("error out"=w407:errorcluster, "value"=w394:dbl, "refnum out"=w406:T10)  [unwired: 4 in, 1 out]
        n252 = local write "浓度2"(w394) -> ()
        n253 = call-poly <vilib>:"Read Key.vi"("section"=w350, "error in (no error)"=w407, "key"="浓度3", "refnum"=w406) -> ("error out"=w408:errorcluster, "value"=w396:dbl, "refnum out"=w405:T10)  [unwired: 4 in, 1 out]
        n254 = local write "浓度3"(w396) -> ()
        n255 = call-poly <vilib>:"Read Key.vi"("section"=w350, "error in (no error)"=w408, "key"="泵滴定数1", "refnum"=w405) -> ("error out"=w409:errorcluster, "value"=w398:dbl, "refnum out"=w404:T10)  [unwired: 4 in, 1 out]
        n256 = local write "泵滴定数1"(w398) -> ()
        n257 = call-poly <vilib>:"Read Key.vi"("section"=w350, "error in (no error)"=w409, "key"="泵滴定数2", "refnum"=w404) -> ("error out"=w403:errorcluster, "value"=w401:dbl, "refnum out"=w410:T10)  [unwired: 4 in, 1 out]
        n258 = local write "泵滴定数2"(w401) -> ()
        n259 = call-poly <vilib>:"Read Key.vi"("section"=w350, "error in (no error)"=w403, "key"="泵滴定数3", "refnum"=w410) -> ("error out"=w418:errorcluster, "value"=w417:dbl, "refnum out"=w411:T10)  [unwired: 4 in, 1 out]
        n260 = local write "泵滴定数3"(w417) -> ()
        n261 = call-poly <vilib>:"Read Key.vi"("section"=w350, "error in (no error)"=w418, "key"="浓度4", "refnum"=w411) -> ("error out"=w419:errorcluster, "value"=w425:dbl, "refnum out"=w412:T10)  [unwired: 4 in, 1 out]
        n262 = local write "浓度4"(w425) -> ()
        n263 = call-poly <vilib>:"Read Key.vi"("section"=w350, "error in (no error)"=w419, "key"="浓度5", "refnum"=w412) -> ("error out"=w420:errorcluster, "value"=w426:dbl, "refnum out"=w413:T10)  [unwired: 4 in, 1 out]
        n264 = local write "浓度5"(w426) -> ()
        n265 = call-poly <vilib>:"Read Key.vi"("section"=w350, "error in (no error)"=w420, "key"="浓度6", "refnum"=w413) -> ("error out"=w421:errorcluster, "value"=w427:dbl, "refnum out"=w414:T10)  [unwired: 4 in, 1 out]
        n266 = local write "浓度6"(w427) -> ()
        n267 = call-poly <vilib>:"Read Key.vi"("section"=w350, "error in (no error)"=w421, "key"="泵滴定数4", "refnum"=w414) -> ("error out"=w422:errorcluster, "value"=w428:dbl, "refnum out"=w415:T10)  [unwired: 4 in, 1 out]
        n268 = local write "泵滴定数4"(w428) -> ()
        n269 = call-poly <vilib>:"Read Key.vi"("section"=w350, "error in (no error)"=w422, "key"="泵滴定数5", "refnum"=w415) -> ("error out"=w423:errorcluster, "value"=w429:dbl, "refnum out"=w416:T10)  [unwired: 4 in, 1 out]
        n270 = local write "泵滴定数5"(w429) -> ()
        n271 = call-poly <vilib>:"Read Key.vi"("section"=w350, "error in (no error)"=w423, "key"="泵滴定数6", "refnum"=w416) -> ("error out"=w381:errorcluster, "value"=w430:dbl, "refnum out"=w384:T10)  [unwired: 4 in, 1 out]
        n272 = local write "泵滴定数6"(w430) -> ()
        n273 = call-poly <vilib>:"Read Key.vi"("section"=w350, "error in (no error)"=w381, "key"="当前选用的校准", "refnum"=w384) -> ("error out"=w379:errorcluster, "value"=w382:i32, "refnum out"=w380:T10)  [unwired: 4 in, 1 out]
        n274 = local write "当前校准"(w382) -> ()
        n275 = call-poly <vilib>:"Read Key.vi"("section"=w350, "error in (no error)"=w379, "key"="启用1", "refnum"=w380) -> ("error out"=w376:errorcluster, "value"=w362:bool, "refnum out"=w377:T10)  [unwired: 4 in, 1 out]
        n276 = local write "启用1"(w362) -> ()
        n277 = call-poly <vilib>:"Read Key.vi"("section"=w350, "error in (no error)"=w376, "key"="启用2", "refnum"=w377) -> ("error out"=w374:errorcluster, "value"=w361:bool, "refnum out"=w375:T10)  [unwired: 4 in, 1 out]
        n278 = local write "启用2"(w361) -> ()
        n279 = call-poly <vilib>:"Read Key.vi"("section"=w350, "error in (no error)"=w374, "key"="启用3", "refnum"=w375) -> ("error out"=w372:errorcluster, "value"=w360:bool, "refnum out"=w373:T10)  [unwired: 4 in, 1 out]
        n280 = local write "启用3"(w360) -> ()
        n281 = call-poly <vilib>:"Read Key.vi"("section"=w350, "error in (no error)"=w372, "key"="启用4", "refnum"=w373) -> ("error out"=w370:errorcluster, "value"=w359:bool, "refnum out"=w371:T10)  [unwired: 4 in, 1 out]
        n282 = local write "启用4"(w359) -> ()
        n283 = call-poly <vilib>:"Read Key.vi"("section"=w350, "error in (no error)"=w370, "key"="启用5", "refnum"=w371) -> ("error out"=w368:errorcluster, "value"=w358:bool, "refnum out"=w369:T10)  [unwired: 4 in, 1 out]
        n284 = local write "启用5"(w358) -> ()
        n285 = call-poly <vilib>:"Read Key.vi"("section"=w350, "error in (no error)"=w368, "key"="启用6", "refnum"=w369) -> ("error out"=w354:errorcluster, "value"=w357:bool, "refnum out"=w355:T10)  [unwired: 4 in, 1 out]
        n286 = local write "启用6"(w357) -> ()
        n287 = call <vilib>:"Close Config Data.vi"("error in (no error)"=w354, "refnum"=w355) -> ()  [unwired: 8 in, 2 out]
      }
      event "量程选择": Value Change {
        (unwired) "选用水样" ("key")
        (unwired) "标线选择" ("section")
        n288 = event-data() -> ()  [unwired: 1 in, 6 out]
        n289 = property on="窗格" class="Pane"("Origin"=T9 {"Horizontal"=0, "Vertical"=1300} ("原点")) -> ()  [unwired: 2 in, 2 out]
        n290 = local read "选用水样"() -> (w445:enum16{"葡萄糖", "草酸钠"})
        n291 = case shown="\"葡萄糖\", 默认" w445 {
          tunnel: ["葡萄糖标线" ("section") "草酸钠标线" ("section")] -> w444
          frame "葡萄糖", Default {
          }
          frame "草酸钠" {
          }
        }
        n292 = case shown="\"高量程\"" "量程选择" {
          tunnel: ["低量程" "高量程"] -> w441
          frame "低量程", Default {
          }
          frame "高量程" {
          }
        }
        n293 = call <vilib>:"Application Directory.vi"() -> ("Application Directory"=w478:path)
        n294 = Build Path(base path=w478, name or relative path="data\\Set.ini" ("名称或相对路径")) -> (appended path=w476:path)
        n295 = call <vilib>:"Open Config Data.vi"("configuration file path"=w476) -> ("error out"=w479:errorcluster, "refnum"=w480:T10)  [unwired: 8 in, 1 out]
        n296 = Concatenate Strings(w444, w441) -> (w443:string)
        n297 = call-poly <vilib>:"Read Key.vi"("section"=w443, "error in (no error)"=w479, "key"="浓度1", "refnum"=w480) -> ("error out"=w484:errorcluster, "value"=w482:dbl, "refnum out"=w483:T10)  [unwired: 4 in, 1 out]
        n298 = local write "浓度1"(w482) -> ()
        n299 = call-poly <vilib>:"Read Key.vi"("section"=w443, "error in (no error)"=w484, "key"="浓度2", "refnum"=w483) -> ("error out"=w498:errorcluster, "value"=w485:dbl, "refnum out"=w497:T10)  [unwired: 4 in, 1 out]
        n300 = local write "浓度2"(w485) -> ()
        n301 = call-poly <vilib>:"Read Key.vi"("section"=w443, "error in (no error)"=w498, "key"="浓度3", "refnum"=w497) -> ("error out"=w499:errorcluster, "value"=w487:dbl, "refnum out"=w496:T10)  [unwired: 4 in, 1 out]
        n302 = local write "浓度3"(w487) -> ()
        n303 = call-poly <vilib>:"Read Key.vi"("section"=w443, "error in (no error)"=w499, "key"="泵滴定数1", "refnum"=w496) -> ("error out"=w500:errorcluster, "value"=w489:dbl, "refnum out"=w495:T10)  [unwired: 4 in, 1 out]
        n304 = local write "泵滴定数1"(w489) -> ()
        n305 = call-poly <vilib>:"Read Key.vi"("section"=w443, "error in (no error)"=w500, "key"="泵滴定数2", "refnum"=w495) -> ("error out"=w494:errorcluster, "value"=w492:dbl, "refnum out"=w501:T10)  [unwired: 4 in, 1 out]
        n306 = local write "泵滴定数2"(w492) -> ()
        n307 = call-poly <vilib>:"Read Key.vi"("section"=w443, "error in (no error)"=w494, "key"="泵滴定数3", "refnum"=w501) -> ("error out"=w509:errorcluster, "value"=w508:dbl, "refnum out"=w502:T10)  [unwired: 4 in, 1 out]
        n308 = local write "泵滴定数3"(w508) -> ()
        n309 = call-poly <vilib>:"Read Key.vi"("section"=w443, "error in (no error)"=w509, "key"="浓度4", "refnum"=w502) -> ("error out"=w510:errorcluster, "value"=w516:dbl, "refnum out"=w503:T10)  [unwired: 4 in, 1 out]
        n310 = local write "浓度4"(w516) -> ()
        n311 = call-poly <vilib>:"Read Key.vi"("section"=w443, "error in (no error)"=w510, "key"="浓度5", "refnum"=w503) -> ("error out"=w511:errorcluster, "value"=w517:dbl, "refnum out"=w504:T10)  [unwired: 4 in, 1 out]
        n312 = local write "浓度5"(w517) -> ()
        n313 = call-poly <vilib>:"Read Key.vi"("section"=w443, "error in (no error)"=w511, "key"="浓度6", "refnum"=w504) -> ("error out"=w512:errorcluster, "value"=w518:dbl, "refnum out"=w505:T10)  [unwired: 4 in, 1 out]
        n314 = local write "浓度6"(w518) -> ()
        n315 = call-poly <vilib>:"Read Key.vi"("section"=w443, "error in (no error)"=w512, "key"="泵滴定数4", "refnum"=w505) -> ("error out"=w513:errorcluster, "value"=w519:dbl, "refnum out"=w506:T10)  [unwired: 4 in, 1 out]
        n316 = local write "泵滴定数4"(w519) -> ()
        n317 = call-poly <vilib>:"Read Key.vi"("section"=w443, "error in (no error)"=w513, "key"="泵滴定数5", "refnum"=w506) -> ("error out"=w514:errorcluster, "value"=w520:dbl, "refnum out"=w507:T10)  [unwired: 4 in, 1 out]
        n318 = local write "泵滴定数5"(w520) -> ()
        n319 = call-poly <vilib>:"Read Key.vi"("section"=w443, "error in (no error)"=w514, "key"="泵滴定数6", "refnum"=w507) -> ("error out"=w472:errorcluster, "value"=w521:dbl, "refnum out"=w475:T10)  [unwired: 4 in, 1 out]
        n320 = local write "泵滴定数6"(w521) -> ()
        n321 = call-poly <vilib>:"Read Key.vi"("section"=w443, "error in (no error)"=w472, "key"="当前选用的校准", "refnum"=w475) -> ("error out"=w470:errorcluster, "value"=w473:i32, "refnum out"=w471:T10)  [unwired: 4 in, 1 out]
        n322 = local write "当前校准"(w473) -> ()
        n323 = call-poly <vilib>:"Read Key.vi"("section"=w443, "error in (no error)"=w470, "key"="启用1", "refnum"=w471) -> ("error out"=w467:errorcluster, "value"=w453:bool, "refnum out"=w468:T10)  [unwired: 4 in, 1 out]
        n324 = local write "启用1"(w453) -> ()
        n325 = call-poly <vilib>:"Read Key.vi"("section"=w443, "error in (no error)"=w467, "key"="启用2", "refnum"=w468) -> ("error out"=w465:errorcluster, "value"=w452:bool, "refnum out"=w466:T10)  [unwired: 4 in, 1 out]
        n326 = local write "启用2"(w452) -> ()
        n327 = call-poly <vilib>:"Read Key.vi"("section"=w443, "error in (no error)"=w465, "key"="启用3", "refnum"=w466) -> ("error out"=w463:errorcluster, "value"=w451:bool, "refnum out"=w464:T10)  [unwired: 4 in, 1 out]
        n328 = local write "启用3"(w451) -> ()
        n329 = call-poly <vilib>:"Read Key.vi"("section"=w443, "error in (no error)"=w463, "key"="启用4", "refnum"=w464) -> ("error out"=w461:errorcluster, "value"=w450:bool, "refnum out"=w462:T10)  [unwired: 4 in, 1 out]
        n330 = local write "启用4"(w450) -> ()
        n331 = call-poly <vilib>:"Read Key.vi"("section"=w443, "error in (no error)"=w461, "key"="启用5", "refnum"=w462) -> ("error out"=w459:errorcluster, "value"=w449:bool, "refnum out"=w460:T10)  [unwired: 4 in, 1 out]
        n332 = local write "启用5"(w449) -> ()
        n333 = call-poly <vilib>:"Read Key.vi"("section"=w443, "error in (no error)"=w459, "key"="启用6", "refnum"=w460) -> ("error out"=w446:errorcluster, "value"=w448:bool, "refnum out"=w447:T10)  [unwired: 4 in, 1 out]
        n334 = local write "启用6"(w448) -> ()
        n335 = call <vilib>:"Close Config Data.vi"("error in (no error)"=w446, "refnum"=w447) -> ()  [unwired: 8 in, 2 out]
      }
      event "周期设置": Value Change {
        n336 = event-data() -> ()  [unwired: 1 in, 6 out]
        n337 = disable-structure shown="禁用" {
          disable-tunnel: [w535 _] -> _
          frame Disabled {
            n338 = call "请输入管理员密码"() -> ("确定"=w535:bool)  [unwired: 17 in, 2 out]
          }
          frame Enabled {
          }
        }
        n339 = call "数字密码键盘.vi"() -> ("NewNumber"=w532:sgl)  [unwired: 1 in]
        n340 = Equal?(x=w532, y=8.0) -> (x = y?=w533:bool)
        n341 = case shown="真" w533 {
          frame False {
            n342 = call "窗口弹出对话框(子VI).vi"("消息"="密码错误") -> ()  [unwired: 10 in, 1 out]
          }
          frame True {
            n343 = call "窗口弹出对话框(子VI).vi"("消息"="登录成功") -> ("true"=w537:bool)  [unwired: 10 in]
            n344 = case shown="真" w537 {
              frame False {
              }
              frame True {
                n345 = property on="窗格" class="Pane"("Origin"=T9 {"Horizontal"=0, "Vertical"=1950} ("原点")) -> ()  [unwired: 2 in, 2 out]
              }
            }
          }
        }
      }
      event "返回": Value Change {
        w542 = "CODMn" ("section")
        n346 = event-data() -> ()  [unwired: 1 in, 6 out]
        n347 = property on="窗格" class="Pane"("Origin"=T9 {"Horizontal"=0, "Vertical"=0} ("原点")) -> ()  [unwired: 2 in, 2 out]
        n348 = call <vilib>:"Application Directory.vi"() -> ("Application Directory"=w618:path)
        n349 = Build Path(base path=w618, name or relative path="data\\Set.ini" ("名称或相对路径")) -> (appended path=w616:path)
        n350 = local write "读取KB值"(FALSE ("读取KB值")) -> ()
        n351 = call <vilib>:"Open Config Data.vi"("configuration file path"=w616) -> ("error out"=w614:errorcluster, "refnum"=w615:T10)  [unwired: 8 in, 1 out]
        n352 = local read "浓度1"() -> (w612:dbl)
        n353 = local read "浓度2"() -> (w596:dbl)
        n354 = call-poly <vilib>:"Write Key.vi"("section"=w542, "error in (no error)"=w614, "value"=w612, "key"="浓度1", "refnum"=w615) -> ("error out"=w611:errorcluster, "refnum out"=w610:T10)  [unwired: 4 in, 1 out]
        n355 = local read "浓度3"() -> (w586:dbl)
        n356 = call-poly <vilib>:"Write Key.vi"("section"=w542, "error in (no error)"=w611, "value"=w596, "key"="浓度2", "refnum"=w610) -> ("error out"=w609:errorcluster, "refnum out"=w608:T10)  [unwired: 4 in, 1 out]
        n357 = local read "泵滴定数1"() -> (w584:dbl)
        n358 = call-poly <vilib>:"Write Key.vi"("section"=w542, "error in (no error)"=w609, "value"=w586, "key"="浓度3", "refnum"=w608) -> ("error out"=w607:errorcluster, "refnum out"=w606:T10)  [unwired: 4 in, 1 out]
        n359 = call-poly <vilib>:"Write Key.vi"("section"=w542, "error in (no error)"=w607, "value"=w584, "key"="泵滴定数1", "refnum"=w606) -> ("error out"=w605:errorcluster, "refnum out"=w604:T10)  [unwired: 4 in, 1 out]
        n360 = local read "泵滴定数2"() -> (w582:dbl)
        n361 = call-poly <vilib>:"Write Key.vi"("section"=w542, "error in (no error)"=w605, "value"=w582, "key"="泵滴定数2", "refnum"=w604) -> ("error out"=w603:errorcluster, "refnum out"=w602:T10)  [unwired: 4 in, 1 out]
        n362 = local read "泵滴定数3"() -> (w580:dbl)
        n363 = local read "浓度4"() -> (w578:dbl)
        n364 = call-poly <vilib>:"Write Key.vi"("section"=w542, "error in (no error)"=w603, "value"=w580, "key"="泵滴定数3", "refnum"=w602) -> ("error out"=w601:errorcluster, "refnum out"=w600:T10)  [unwired: 4 in, 1 out]
        n365 = local read "浓度5"() -> (w575:dbl)
        n366 = call-poly <vilib>:"Write Key.vi"("section"=w542, "error in (no error)"=w601, "value"=w578, "key"="浓度4", "refnum"=w600) -> ("error out"=w594:errorcluster, "refnum out"=w595:T10)  [unwired: 4 in, 1 out]
        n367 = local read "浓度6"() -> (w574:dbl)
        n368 = call-poly <vilib>:"Write Key.vi"("section"=w542, "error in (no error)"=w594, "value"=w575, "key"="浓度5", "refnum"=w595) -> ("error out"=w593:errorcluster, "refnum out"=w592:T10)  [unwired: 4 in, 1 out]
        n369 = call-poly <vilib>:"Write Key.vi"("section"=w542, "error in (no error)"=w593, "value"=w574, "key"="浓度6", "refnum"=w592) -> ("error out"=w590:errorcluster, "refnum out"=w591:T10)  [unwired: 4 in, 1 out]
        n370 = local read "泵滴定数4"() -> (w572:dbl)
        n371 = call-poly <vilib>:"Write Key.vi"("section"=w542, "error in (no error)"=w590, "value"=w572, "key"="泵滴定数4", "refnum"=w591) -> ("error out"=w599:errorcluster, "refnum out"=w598:T10)  [unwired: 4 in, 1 out]
        n372 = local read "泵滴定数5"() -> (w570:dbl)
        n373 = call-poly <vilib>:"Write Key.vi"("section"=w542, "error in (no error)"=w599, "value"=w570, "key"="泵滴定数5", "refnum"=w598) -> ("error out"=w588:errorcluster, "refnum out"=w589:T10)  [unwired: 4 in, 1 out]
        n374 = local read "泵滴定数6"() -> (w568:dbl)
        n375 = local read "启用1"() -> (w558:bool)
        n376 = call-poly <vilib>:"Write Key.vi"("section"=w542, "error in (no error)"=w588, "value"=w568, "key"="泵滴定数6", "refnum"=w589) -> ("error out"=w567:errorcluster, "refnum out"=w566:T10)  [unwired: 4 in, 1 out]
        n377 = call-poly <vilib>:"Write Key.vi"("section"=w542, "error in (no error)"=w567, "value"=w558, "key"="启用1", "refnum"=w566) -> ("error out"=w554:errorcluster, "refnum out"=w557:T10)  [unwired: 4 in, 1 out]
        n378 = local read "启用2"() -> (w555:bool)
        n379 = call-poly <vilib>:"Write Key.vi"("section"=w542, "error in (no error)"=w554, "value"=w555, "key"="启用2", "refnum"=w557) -> ("error out"=w565:errorcluster, "refnum out"=w564:T10)  [unwired: 4 in, 1 out]
        n380 = local read "启用3"() -> (w553:bool)
        n381 = local read "启用4"() -> (w551:bool)
        n382 = call-poly <vilib>:"Write Key.vi"("section"=w542, "error in (no error)"=w565, "value"=w553, "key"="启用3", "refnum"=w564) -> ("error out"=w563:errorcluster, "refnum out"=w562:T10)  [unwired: 4 in, 1 out]
        n383 = local read "启用5"() -> (w548:bool)
        n384 = call-poly <vilib>:"Write Key.vi"("section"=w542, "error in (no error)"=w563, "value"=w551, "key"="启用4", "refnum"=w562) -> ("error out"=w561:errorcluster, "refnum out"=w560:T10)  [unwired: 4 in, 1 out]
        n385 = call-poly <vilib>:"Write Key.vi"("section"=w542, "error in (no error)"=w561, "value"=w548, "key"="启用5", "refnum"=w560) -> ("error out"=w546:errorcluster, "refnum out"=w545:T10)  [unwired: 4 in, 1 out]
        n386 = local read "启用6"() -> (w547:bool)
        n387 = call-poly <vilib>:"Write Key.vi"("section"=w542, "error in (no error)"=w546, "value"=w547, "key"="启用6", "refnum"=w545) -> ("error out"=w543:errorcluster, "refnum out"=w544:T10)  [unwired: 4 in, 1 out]
        n388 = call <vilib>:"Close Config Data.vi"("error in (no error)"=w543, "refnum"=w544) -> ()  [unwired: 8 in, 2 out]
      }
      event "关闭", "关闭 2": Value Change {
        n389 = event-data() -> ()  [unwired: 1 in, 6 out]
        n390 = property on="窗格" class="Pane"("Origin"=T9 {"Horizontal"=0, "Vertical"=0} ("原点")) -> ()  [unwired: 2 in, 2 out]
      }
      event Timeout; Application Instance Close {
        n391 = event-data() -> ()  [unwired: 1 in, 3 out]
        n392 = call-dynamic "Close Session.vi"("error in (no error)"=w621, "MB_Serial session"=w622) -> ()  [unwired: 9 in, 1 out]
      }
      event "时间校准": Value Change {
        n393 = event-data() -> ()  [unwired: 1 in, 6 out]
        n394 = flat-sequence {
          tunnel: w623 -> [w628]
          frame #0 {
            n395 = Get Date/Time In Seconds() -> (seconds since 1Jan1904=w633:timestamp)
            n396 = Build Array(w633) -> (w632:timestamp[])
            n397 = call "DateToHex.vi"("DATE"=w632) -> ("数组"=w626:u16[])  [unwired: 10 in]
            n398 = Insert Into Array(array=u16[] [1] ("values"), index=1 ("索引"), new element=w626) -> (w624:u16[])
            n399 = Bundle By Name(cluster=cluster{"starting address":u16, "values":u16[]} {"starting address"=0, "values"=[]}, "starting address"=u16 4612, "values"=w624) -> (w629:cluster{"starting address":u16, "values":u16[]})
            n400 = Enqueue Element(queue=w628, element=w629) -> ()  [unwired: 2 in, 3 out]
          }
          frame #1 {
            n401 = local write "枚举"(enum16{"读取数据", "写入数据", "读取写入DATABASE", "读取参数"}."写入数据" ("枚举")) -> ()
          }
        }
      }
      event "故障清除": Value Change {
        n402 = event-data() -> ()  [unwired: 1 in, 6 out]
        n403 = local write "枚举"(enum16{"读取数据", "写入数据", "读取写入DATABASE", "读取参数"}."写入数据" ("枚举")) -> ()
        n404 = Bundle By Name(cluster=cluster{"starting address":u16, "values":u16[]} {"starting address"=0, "values"=[]}, "starting address"=u16 4611, "values"=u16[] [1]) -> (w638:cluster{"starting address":u16, "values":u16[]})
        n405 = Enqueue Element(queue=w637, element=w638) -> ()  [unwired: 2 in, 3 out]
      }
      event "定时启动": Value Change {
        n406 = event-data() -> ()  [unwired: 1 in, 6 out]
        n407 = call "COD定时启动对话框.vi"() -> ("设置值"=→"定时时间":dbl, "确定输出"=w641:bool)  [unwired: 10 in]
        n408 = local write "定时启动"(w641) -> ()
      }
      event "校准1", "校准2", "校准3", "校准4", "校准5", "校准6": Value Change {
        n409 = event-data() -> ()  [unwired: 1 in, 6 out]
        n410 = flat-sequence {
          tunnel: w645 -> [w648]
          tunnel: [w647] -> w644
          tunnel: [w646] -> w643
          tunnel: w644 -> [w685]
          tunnel: w643 -> [w684]
          frame #0 {
            n411 = Build Array("校准1", "校准2", "校准3", "校准4", "校准5", "校准6") -> (w649:bool[])
            n412 = for {
              tunnel: w649 -> [w666] mode=indexing
              tunnel: w648 -> [w662]
              tunnel: [w658] -> w647
              tunnel: [w657] -> w646
              i -> [w656]
              n413 = case shown="3" w656 {
                tunnel: ["浓度1" "浓度2" "浓度3" "浓度4" "浓度5" "浓度6"] -> w661
                frame 0, Default {
                }
                frame 1 {
                }
                frame 2 {
                }
                frame 3 {
                }
                frame 4 {
                }
                frame 5 {
                }
              }
              n414 = Multiply(x=w661, y=100.0) -> (x*y=w659:dbl)
              n415 = Insert Into Array(array=u16[] [] ("values"), index=0 ("索引"), new element=w659) -> (w663:u16[])
              n416 = case shown="真" w666 {
                tunnel: w663 -> [_ w679]
                tunnel: w662 -> [w673 w678]
                tunnel: [w673 w677] -> w658
                tunnel: [_ w676] -> w657
                tunnel: w656 -> [_ w675]
                frame False {
                }
                frame True {
                  n417 = Increment(x=w675) -> (x+1=→"当前校准":i32)
                  n418 = Bundle By Name(cluster=cluster{"starting address":u16, "values":u16[]} {"starting address"=4272, "values"=[]}, "starting address"=u16 4274, "values"=w679) -> (w681:cluster{"starting address":u16, "values":u16[]})
                  n419 = Enqueue Element(queue=w678, element=w681) -> (queue out=w677:refnum<queue>, error out=w676:errorcluster)  [unwired: 2 in, 1 out]
                }
              }
            }
          }
          frame #1 {
            n420 = local read "当前校准"() -> (w690:i32)
            n421 = case shown="4" w690 {
              tunnel: [w696 w697 w698 w699 w700 w701] -> w689
              frame 1, Default {
                n422 = local read "浓度1"() -> (w696:dbl)
              }
              frame 2 {
                n423 = local read "浓度2"() -> (w697:dbl)
              }
              frame 3 {
                n424 = local read "浓度3"() -> (w698:dbl)
              }
              frame 4 {
                n425 = local read "浓度4"() -> (w699:dbl)
              }
              frame 5 {
                n426 = local read "浓度5"() -> (w700:dbl)
              }
              frame 6 {
                n427 = local read "浓度6"() -> (w701:dbl)
              }
            }
            n428 = Not Equal To 0?(x=w689) -> (x != 0?=w688:bool)
            n429 = case shown="真" w688 {
              tunnel: [u16 8 ("address") u16 9 ("address")] -> w693
              tunnel: ["校零" ("测量模式") "校标" ("测量模式")] -> w683
              frame False {
              }
              frame True {
              }
            }
            n430 = global write "COD测量模式全局.vi" "测量模式"(w683) -> ()
            n431 = Insert Into Array(array=u16[] [] ("values"), index=0 ("索引"), new element=w693) -> (w687:u16[])
            n432 = Bundle By Name(cluster=cluster{"starting address":u16, "values":u16[]} {"starting address"=0, "values"=[]}, "starting address"=u16 4608 ("address"), "values"=w687) -> (w695:cluster{"starting address":u16, "values":u16[]})
            n433 = Enqueue Element(queue=w685, element=w695, error in (no error)=w684) -> ()  [unwired: 1 in, 3 out]
          }
          frame #2 {
            n434 = local write "枚举"(enum16{"读取数据", "写入数据", "读取写入DATABASE", "读取参数"}."写入数据" ("枚举")) -> ()
            n435 = call <vilib>:"Application Directory.vi"() -> ("Application Directory"=w713:path)
            n436 = Build Path(base path=w713, name or relative path="data\\Set.ini" ("名称或相对路径")) -> (appended path=w715:path)
            n437 = local read "当前校准"() -> (w708:i32)
            n438 = call <vilib>:"Open Config Data.vi"("configuration file path"=w715) -> ("error out"=w711:errorcluster, "refnum"=w712:T10)  [unwired: 8 in, 1 out]
            n439 = call-poly <vilib>:"Write Key.vi"("section"="CODMn", "error in (no error)"=w711, "value"=w708, "key"="当前选用的校准" ("section"), "refnum"=w712) -> ("error out"=w706:errorcluster, "refnum out"=w707:T10)  [unwired: 4 in, 1 out]
            n440 = call <vilib>:"Close Config Data.vi"("error in (no error)"=w706, "refnum"=w707) -> ()  [unwired: 8 in, 2 out]
          }
        }
      }
      event "自动切换量程": Value Change {
        n441 = event-data() -> ()  [unwired: 1 in, 6 out]
        n442 = call <vilib>:"Application Directory.vi"() -> ("Application Directory"=w726:path)
        n443 = Build Path(base path=w726, name or relative path="data\\Set.ini" ("名称或相对路径")) -> (appended path=w724:path)
        n444 = local read "自动切换量程"() -> (w719:bool)
        n445 = call <vilib>:"Open Config Data.vi"("configuration file path"=w724) -> ("error out"=w722:errorcluster, "refnum"=w723:T10)  [unwired: 8 in, 1 out]
        n446 = call-poly <vilib>:"Write Key.vi"("section"="CODMn是否切换量程" ("key"), "error in (no error)"=w722, "value"=w719, "key"="自动切换量程", "refnum"=w723) -> ("error out"=w717:errorcluster, "refnum out"=w718:T10)  [unwired: 4 in, 1 out]
        n447 = call <vilib>:"Close Config Data.vi"("error in (no error)"=w717, "refnum"=w718) -> ()  [unwired: 8 in, 2 out]
      }
      event "模型": Value Change {
        n448 = event-data() -> ()  [unwired: 1 in, 6 out]
        n449 = call <vilib>:"Application Directory.vi"() -> ("Application Directory"=w736:path)
        n450 = Build Path(base path=w736, name or relative path="data\\Set.ini" ("名称或相对路径")) -> (appended path=w734:path)
        n451 = call <vilib>:"Open Config Data.vi"("configuration file path"=w734) -> ("error out"=w732:errorcluster, "refnum"=w733:T10)  [unwired: 8 in, 1 out]
        n452 = local read "模型"() -> (w727:enum32{"线性", "多项式"})
        n453 = call-poly <vilib>:"Write Key.vi"("section"="CODMn模型选择" ("key"), "error in (no error)"=w732, "value"=w727, "key"="线性和多项式", "refnum"=w733) -> ("error out"=w728:errorcluster, "refnum out"=w729:T10)  [unwired: 4 in, 1 out]
        n454 = call <vilib>:"Close Config Data.vi"("error in (no error)"=w728, "refnum"=w729) -> ()  [unwired: 8 in, 2 out]
      }
      event "浓度1", "浓度2", "浓度3", "泵滴定数1", "泵滴定数2", "泵滴定数3", "浓度4", "浓度5", "浓度6", "泵滴定数4", "泵滴定数5", "泵滴定数6", "启用1", "启用2", "启用3", "启用4", "启用5", "启用6": Value Change {
        n455 = event-data() -> ()  [unwired: 1 in, 6 out]
        n456 = local read "选用水样"() -> (w740:enum16{"葡萄糖", "草酸钠"})
        n457 = local read "量程选择"() -> (w739:enum16{"低量程", "高量程"})
        n458 = case shown="\"高量程\"" w739 {
          tunnel: ["低量程" "高量程"] -> w737
          frame "低量程", Default {
          }
          frame "高量程" {
          }
        }
        n459 = call <vilib>:"Application Directory.vi"() -> ("Application Directory"=w823:path)
        n460 = case shown="\"葡萄糖\", 默认" w740 {
          tunnel: ["葡萄糖标线" ("section") "草酸钠标线" ("section")] -> w746
          frame "葡萄糖", Default {
          }
          frame "草酸钠" {
          }
        }
        n461 = Build Path(base path=w823, name or relative path="data\\Set.ini" ("名称或相对路径")) -> (appended path=w821:path)
        n462 = call <vilib>:"Open Config Data.vi"("configuration file path"=w821) -> ("error out"=w819:errorcluster, "refnum"=w820:T10)  [unwired: 8 in, 1 out]
        n463 = local read "浓度1"() -> (w817:dbl)
        n464 = Concatenate Strings(w746, w737) -> (w738:string)
        n465 = local read "浓度2"() -> (w801:dbl)
        n466 = call-poly <vilib>:"Write Key.vi"("section"=w738, "error in (no error)"=w819, "value"=w817, "key"="浓度1", "refnum"=w820) -> ("error out"=w816:errorcluster, "refnum out"=w815:T10)  [unwired: 4 in, 1 out]
        n467 = local read "浓度3"() -> (w791:dbl)
        n468 = call-poly <vilib>:"Write Key.vi"("section"=w738, "error in (no error)"=w816, "value"=w801, "key"="浓度2", "refnum"=w815) -> ("error out"=w814:errorcluster, "refnum out"=w813:T10)  [unwired: 4 in, 1 out]
        n469 = local read "泵滴定数1"() -> (w789:dbl)
        n470 = call-poly <vilib>:"Write Key.vi"("section"=w738, "error in (no error)"=w814, "value"=w791, "key"="浓度3", "refnum"=w813) -> ("error out"=w812:errorcluster, "refnum out"=w811:T10)  [unwired: 4 in, 1 out]
        n471 = call-poly <vilib>:"Write Key.vi"("section"=w738, "error in (no error)"=w812, "value"=w789, "key"="泵滴定数1", "refnum"=w811) -> ("error out"=w810:errorcluster, "refnum out"=w809:T10)  [unwired: 4 in, 1 out]
        n472 = local read "泵滴定数2"() -> (w787:dbl)
        n473 = call-poly <vilib>:"Write Key.vi"("section"=w738, "error in (no error)"=w810, "value"=w787, "key"="泵滴定数2", "refnum"=w809) -> ("error out"=w808:errorcluster, "refnum out"=w807:T10)  [unwired: 4 in, 1 out]
        n474 = local read "泵滴定数3"() -> (w785:dbl)
        n475 = local read "浓度4"() -> (w783:dbl)
        n476 = call-poly <vilib>:"Write Key.vi"("section"=w738, "error in (no error)"=w808, "value"=w785, "key"="泵滴定数3", "refnum"=w807) -> ("error out"=w806:errorcluster, "refnum out"=w805:T10)  [unwired: 4 in, 1 out]
        n477 = local read "浓度5"() -> (w780:dbl)
        n478 = call-poly <vilib>:"Write Key.vi"("section"=w738, "error in (no error)"=w806, "value"=w783, "key"="浓度4", "refnum"=w805) -> ("error out"=w799:errorcluster, "refnum out"=w800:T10)  [unwired: 4 in, 1 out]
        n479 = local read "浓度6"() -> (w779:dbl)
        n480 = call-poly <vilib>:"Write Key.vi"("section"=w738, "error in (no error)"=w799, "value"=w780, "key"="浓度5", "refnum"=w800) -> ("error out"=w798:errorcluster, "refnum out"=w797:T10)  [unwired: 4 in, 1 out]
        n481 = call-poly <vilib>:"Write Key.vi"("section"=w738, "error in (no error)"=w798, "value"=w779, "key"="浓度6", "refnum"=w797) -> ("error out"=w795:errorcluster, "refnum out"=w796:T10)  [unwired: 4 in, 1 out]
        n482 = local read "泵滴定数4"() -> (w777:dbl)
        n483 = call-poly <vilib>:"Write Key.vi"("section"=w738, "error in (no error)"=w795, "value"=w777, "key"="泵滴定数4", "refnum"=w796) -> ("error out"=w804:errorcluster, "refnum out"=w803:T10)  [unwired: 4 in, 1 out]
        n484 = local read "泵滴定数5"() -> (w775:dbl)
        n485 = call-poly <vilib>:"Write Key.vi"("section"=w738, "error in (no error)"=w804, "value"=w775, "key"="泵滴定数5", "refnum"=w803) -> ("error out"=w793:errorcluster, "refnum out"=w794:T10)  [unwired: 4 in, 1 out]
        n486 = local read "泵滴定数6"() -> (w773:dbl)
        n487 = local read "启用1"() -> (w763:bool)
        n488 = call-poly <vilib>:"Write Key.vi"("section"=w738, "error in (no error)"=w793, "value"=w773, "key"="泵滴定数6", "refnum"=w794) -> ("error out"=w772:errorcluster, "refnum out"=w771:T10)  [unwired: 4 in, 1 out]
        n489 = call-poly <vilib>:"Write Key.vi"("section"=w738, "error in (no error)"=w772, "value"=w763, "key"="启用1", "refnum"=w771) -> ("error out"=w759:errorcluster, "refnum out"=w762:T10)  [unwired: 4 in, 1 out]
        n490 = local read "启用2"() -> (w760:bool)
        n491 = call-poly <vilib>:"Write Key.vi"("section"=w738, "error in (no error)"=w759, "value"=w760, "key"="启用2", "refnum"=w762) -> ("error out"=w770:errorcluster, "refnum out"=w769:T10)  [unwired: 4 in, 1 out]
        n492 = local read "启用3"() -> (w758:bool)
        n493 = local read "启用4"() -> (w756:bool)
        n494 = call-poly <vilib>:"Write Key.vi"("section"=w738, "error in (no error)"=w770, "value"=w758, "key"="启用3", "refnum"=w769) -> ("error out"=w768:errorcluster, "refnum out"=w767:T10)  [unwired: 4 in, 1 out]
        n495 = call-poly <vilib>:"Write Key.vi"("section"=w738, "error in (no error)"=w768, "value"=w756, "key"="启用4", "refnum"=w767) -> ("error out"=w766:errorcluster, "refnum out"=w765:T10)  [unwired: 4 in, 1 out]
        n496 = local read "启用5"() -> (w753:bool)
        n497 = call-poly <vilib>:"Write Key.vi"("section"=w738, "error in (no error)"=w766, "value"=w753, "key"="启用5", "refnum"=w765) -> ("error out"=w751:errorcluster, "refnum out"=w750:T10)  [unwired: 4 in, 1 out]
        n498 = local read "启用6"() -> (w752:bool)
        n499 = call-poly <vilib>:"Write Key.vi"("section"=w738, "error in (no error)"=w751, "value"=w752, "key"="启用6", "refnum"=w750) -> ("error out"=w747:errorcluster, "refnum out"=w748:T10)  [unwired: 4 in, 1 out]
        n500 = local read "选用水样"() -> (w745:enum16{"葡萄糖", "草酸钠"})
        n501 = call-poly <vilib>:"Write Key.vi"("section"="标线选择", "error in (no error)"=w747, "value"=w745, "key"="选用水样", "refnum"=w748) -> ("error out"=w742:errorcluster, "refnum out"=w743:T10)  [unwired: 4 in, 1 out]
        n502 = call <vilib>:"Close Config Data.vi"("error in (no error)"=w742, "refnum"=w743) -> ()  [unwired: 8 in, 2 out]
      }
      event "读取": Value Change {
        n503 = event-data() -> ()  [unwired: 1 in, 6 out]
        n504 = local write "枚举"(enum16{"读取数据", "写入数据", "读取写入DATABASE", "读取参数"}."读取参数" ("枚举")) -> ()
        n505 = Bundle By Name(cluster=T6 {"starting address"=0, "number of holding registers"=0}, "starting address"=u16 4616, "number of holding registers"=u16 22) -> (w837:T6)
        n506 = Flush Queue(queue=w830, error in (no error)=w829) -> (queue out=w833:refnum<queue>, error out=w832:errorcluster)  [unwired: 1 out]
        n507 = Enqueue Element(queue=w833, element=w837, error in (no error)=w832) -> ()  [unwired: 1 in, 3 out]
        "读取KB值" <- TRUE
      }
      event "写入": Mouse Down {
        n508 = event-data() -> ()  [unwired: 1 in, 8 out]
        n509 = flat-sequence {
          tunnel: w838 -> [w841]
          frame #0 {
            n510 = local read "模型"() -> (w839:enum32{"线性", "多项式"})
            n511 = case shown="\"多项式\"" w839 {
              tunnel: [w853 w859] -> w843
              tunnel: w841 -> [w847 w858]
              tunnel: [w847 w858] -> w840
              frame "线性", Default {
                n512 = local read "K"() -> (w850:dbl)
                n513 = local read "b"() -> (w849:dbl)
                n514 = Build Array(w850, w849, 0.0 ("元素")) -> (w848:dbl[])
                n515 = local read "量程选择"() -> (w846:enum16{"低量程", "高量程"})
                n516 = call "浮点转CDAB整形cod.vi"("浮点数"=w848) -> ("CDAB整形输出"=w851:u16[])  [unwired: 10 in]
                n517 = case shown="\"低量程\", 默认" w846 {
                  tunnel: [u16 4626 ("starting address") u16 4632 ("starting address")] -> w845
                  frame "低量程", Default {
                  }
                  frame "高量程" {
                  }
                }
                n518 = Bundle By Name(cluster=cluster{"starting address":u16, "values":u16[]} {"starting address"=4272, "values"=[]}, "starting address"=w845, "values"=w851) -> (w853:cluster{"starting address":u16, "values":u16[]})
              }
              frame "多项式" {
                # "b,k,c"
                n519 = local read "多项式系数1"() -> (w866:dbl[])
                n520 = local read "量程选择"() -> (w856:enum16{"低量程", "高量程"})
                n521 = Index Array(array=w866) -> (element #1=w861:dbl, element #2=w862:dbl, element #3=w857:dbl)  [unwired: 3 in]
                n522 = Build Array(w862, w861, w857) -> (w865:dbl[])
                n523 = case shown="\"低量程\", 默认" w856 {
                  tunnel: [u16 4626 ("starting address") u16 4632 ("starting address")] -> w863
                  frame "低量程", Default {
                  }
                  frame "高量程" {
                  }
                }
                n524 = call "浮点转CDAB整形cod.vi"("浮点数"=w865) -> ("CDAB整形输出"=w864:u16[])  [unwired: 10 in]
                n525 = Bundle By Name(cluster=cluster{"starting address":u16, "values":u16[]} {"starting address"=4272, "values"=[]}, "starting address"=w863, "values"=w864) -> (w859:cluster{"starting address":u16, "values":u16[]})
              }
            }
            n526 = Enqueue Element(queue=w840, element=w843, timeout in ms (-1)=1000 ("超时毫秒(-1)")) -> ()  [unwired: 1 in, 3 out]
          }
          frame #1 {
            n527 = local write "枚举"(enum16{"读取数据", "写入数据", "读取写入DATABASE", "读取参数"}."写入数据" ("枚举")) -> ()
          }
        }
      }
    }
  }
  n528 = while {
    tunnel: w23 -> [w999]
    tunnel: w22 -> [w998]
    tunnel: w11 -> [w993]
    tunnel: w10 -> [w992]
    i -> [w994]
    stop <- FALSE stop-if-true
    w889 = T12 0 items=["最小二乘", "最小绝对残差", "Bisquare"] ("method")
    w898 = T12 0 items=["最小二乘", "最小绝对残差", "Bisquare"] ("method")
    # "自动校时"
    n529 = Multiply(x="浓度 2", y=100.0) -> (x*y=w963:dbl)
    n530 = Multiply(x="温度", y=10.0) -> (x*y=w966:dbl)
    n531 = local read "启用3"() -> (w918:bool)
    n532 = Wait (ms)(milliseconds to wait=u32 1000 ("等待时间（毫秒）")) -> ()  [unwired: 1 out]
    n533 = local read "启用2"() -> (w917:bool)
    n534 = local read "泵滴定数3"() -> (w915:dbl)
    n535 = local read "泵滴定数1"() -> (w913:dbl)
    n536 = local read "泵滴定数2"() -> (w914:dbl)
    n537 = local read "启用1"() -> (w916:bool)
    n538 = local read "启用6"() -> (w919:bool)
    n539 = local read "启用5"() -> (w920:bool)
    n540 = local read "泵滴定数6"() -> (w922:dbl)
    n541 = local read "泵滴定数4"() -> (w924:dbl)
    n542 = local read "泵滴定数5"() -> (w923:dbl)
    n543 = local read "启用4"() -> (w921:bool)
    n544 = local read "浓度2"() -> (w911:dbl)
    n545 = local read "浓度3"() -> (w912:dbl)
    n546 = local read "浓度1"() -> (w910:dbl)
    n547 = local write "浓度"(w963) -> ()
    n548 = local read "浓度5"() -> (w926:dbl)
    n549 = local read "浓度6"() -> (w925:dbl)
    n550 = local read "浓度4"() -> (w927:dbl)
    n551 = local write "温度 2"(w966) -> ()
    n552 = Bundle By Name(cluster=T6 {"starting address"=4224, "number of holding registers"=16}, "starting address"=u16 4224, "number of holding registers"=u16 50) -> (w1054:T6)
    n553 = Multiply(x="修正系数 2", y=100.0) -> (x*y=w960:dbl)
    n554 = local read "模型"() -> (w879:enum32{"线性", "多项式"})
    n555 = Build Array(w916, w917, w918) -> (w899:bool[])
    n556 = Build Array(w921, w920, w919) -> (w888:bool[])
    n557 = Build Array(w910, w911, w912) -> (w901:dbl[])
    n558 = local write "修正系数"(w960) -> ()
    n559 = Build Array(w913, w914, w915) -> (w900:dbl[])
    n560 = Build Array(w927, w926, w925) -> (w891:dbl[])
    n561 = Build Array(w924, w923, w922) -> (w890:dbl[])
    n562 = call "线性公式CODMn用.vi"("标液浓度"=w901, "监测浓度"=w900, "启用"=w899, "method"=w898, "模型"="模型", "精度"=4) -> ("拟合方程"=→"拟合公式":string, "r^2"=→"r^2":dbl, "slope"=→"K":dbl, "intercept"=→"b":dbl, "XY图"=→"XY图":cluster{"X Values":dbl[], "Y Values":dbl[]}[], "Polynomial Coefficients"=→"多项式系数1":dbl[])  [unwired: 8 in]
    n563 = call "线性公式CODMn用.vi"("标液浓度"=w891, "监测浓度"=w890, "启用"=w888, "method"=w889, "模型"=w879, "精度"=4) -> ("拟合方程"=→"高量程拟合方程":string, "r^2"=→"r^2":dbl, "slope"=→"K 2":dbl, "intercept"=→"b 2":dbl, "XY图"=→"XY图 2":cluster{"X Values":dbl[], "Y Values":dbl[]}[], "Polynomial Coefficients"=→"多项式系数2":dbl[])  [unwired: 8 in]
    n564 = disable-structure shown="禁用" {
      frame Disabled {
        n565 = global read "系统变量.vi" "自动切换量程"() -> (w1055:bool)
        n566 = local write "自动切换量程"(w1055) -> ()
      }
      frame Enabled {
      }
    }
    n567 = Enqueue Element(queue=w999, element=w1054, error in (no error)=w998) -> ()  [unwired: 1 in, 3 out]
    n568 = local read "Registers"() -> (w878:u16[])
    n569 = To Word Integer(number=w878) -> (16bit integer=w877:i16[])
    n570 = Index Array(array=w877, index #1=0 ("索引"), index #4=3 ("索引"), index #14=13 ("索引"), index #15=14 ("索引"), index #32=31 ("索引")) -> (element #1=w957:i16, element #2=w956:i16, element #3=w955:i16, element #4=w872:i16, element #5=→"模式（受控）":i16, element #6=→"进样管":i16, element #7=→"高锰酸钾":i16, element #8=→"草酸钠":i16, element #9=→"硫酸":i16, element #10=w876:i16, element #11=w1026:i16, element #12=w1028:i16, element #13=w1041:i16, element #14=w1045:i16, element #15=w1001:i16, element #16=w904:i16, element #33=→"分":i16, element #34=→"秒":i16)  [unwired: 29 in, 16 out]
    "多列列表框" <- w904
    n571 = To Single Precision Float(number=w876) -> (single precision float=→"ORP显示":sgl)
    n572 = Divide(x=w1045, y=u16 1000) -> (x/y=→"零点滴定值":dbl)
    n573 = Divide(x=w1001, y=u16 1000) -> (x/y=→"标度滴定值":dbl)
    n574 = global write "运行时序全局变量.vi" "多列列表框"(w904) -> ()
    n575 = feedback #1(w904) -> (w973:i16)
    n576 = feedback-in #1(w904) -> ()
    n577 = Build Array(w957, w956, w955) -> (w958:i16[])
    n578 = Equal?(x=w1028, y=u16 1) -> (x = y?=→"排液标记":bool)
    n579 = Equal?(x=w872, y=u16 0) -> (x = y?=→"待机":bool)
    n580 = Equal?(x=w872, y=u16 7) -> (x = y?=→"质控样测量":bool)
    n581 = Equal?(x=w872, y=u16 1) -> (x = y?=→"水样测量":bool)
    n582 = Equal?(x=w904, y=u16 5) -> (x = y?=w997:bool)
    n583 = Equal?(x=w872, y=u16 9) -> (x = y?=→"校标标记":bool)
    n584 = Equal?(x=w872, y=u16 6) -> (x = y?=→"平行样测量":bool)
    n585 = Equal?(x=w872, y=u16 2) -> (x = y?=→"标样核查标记":bool)
    n586 = Equal?(x=w872, y=u16 8) -> (x = y?=→"校零标记":bool)
    n587 = Equal?(x=w1041, y=u16 1) -> (x = y?=w990:bool)
    "ORP故障" <- w990
    n588 = Equal?(x=w1041, y=u16 2) -> (x = y?=w989:bool)
    "温控器故障" <- w989
    n589 = Equal?(x=w1041, y=u16 3) -> (x = y?=w988:bool)
    "加热故障" <- w988
    n590 = Equal?(x=w1041, y=u16 4) -> (x = y?=w987:bool)
    "高锰酸钾报警" <- w987
    n591 = Equal?(x=w1041, y=u16 5) -> (x = y?=w986:bool)
    "草酸钠报警" <- w986
    n592 = Equal?(x=w1041, y=u16 6) -> (x = y?=w985:bool)
    "测量错误" <- w985
    n593 = Equal?(x=w1041, y=u16 8) -> (x = y?=w984:bool)
    "校零错误" <- w984
    n594 = Equal?(x=w1041, y=u16 7) -> (x = y?=w983:bool)
    "校标错误" <- w983
    n595 = Equal?(x=w1041, y=u16 9) -> (x = y?=w982:bool)
    "进水样超量程" <- w982
    n596 = Divide(x=w1026, y=u16 10) -> (x/y=→"温度":dbl)
    n597 = Equal?(x=w872, y=u16 10) -> (x = y?=→"加标回收测量":bool)
    n598 = Equal?(x=w1041, y=u16 10) -> (x = y?=w981:bool)
    "排液故障" <- w981
    n599 = Compound Arithmetic op=OR ("复合运算")(w990, w989, w988, w987, w986, w985, w983, w984, w982, w981) -> (→"故障标记":bool)
    n600 = Not Equal?(x=w904, y=w973) -> (x != y?=w972:bool)
    n601 = call <vilib>:"Boolean Crossing PtByPt.vi"("direction"=enum16{"either", "false-true", "true-false"}."false-true", "input"=w997) -> ("crossing"=w995:bool)  [unwired: 1 in]
    n602 = Bundle By Name(cluster=T3 {"ORP故障"=FALSE, "温控器故障"=FALSE, "加热故障"=FALSE, "高锰酸钾报警"=FALSE, "草酸钠报警"=FALSE, "测量错误"=FALSE, "校零错误"=FALSE, "校标错误"=FALSE, " 进水样超量程"=FALSE, "排液阀故障"=FALSE} ("报警簇"), "ORP故障"=w990, "温控器故障"=w989, "加热故障"=w988, "高锰酸钾报警"=w987, "草酸钠报警"=w986, "测量错误"=w985, "校零错误"=w984, "校标错误"=w983, "进水样超量程"=w982, "排液阀故障"=w981) -> (w974:T3)
    "报警簇" <- w974
    n603 = call "HexToDate.vi"("数组"=w958) -> ("DATE"=w953:timestamp[])  [unwired: 10 in]
    n604 = Equal?(x=w872, y=u16 3) -> (x = y?=→"零点核查标记":bool)
    n605 = Equal?(x=w872, y=u16 4) -> (x = y?=→"跨度核查标记":bool)
    n606 = Equal?(x=w872, y=u16 5) -> (x = y?=→"空白测试标记":bool)
    n607 = case shown="真" w995 {
      tunnel: w993 -> [_ w1157]
      tunnel: w992 -> [_ w1152]
      frame False {
      }
      frame True {
        n608 = Bundle By Name(cluster=T6 {"starting address"=0, "number of holding registers"=0}, "starting address"=u16 4101, "number of holding registers"=u16 10) -> (w1156:T6)
        n609 = Enqueue Element(queue=w1157, element=w1156, error in (no error)=w1152) -> ()  [unwired: 1 in, 3 out]
        n610 = local write "枚举"(enum16{"读取数据", "写入数据", "读取写入DATABASE", "读取参数"}."读取写入DATABASE" ("枚举")) -> ()
      }
    }
    n611 = case shown="真" w972 {
      tunnel: w904 -> [_ w1135]
      frame False {
      }
      frame True {
        n612 = property on="多列列表框" class="MCListbox (严格)"() -> ("ItemNames"=w1129:string[][])  [unwired: 2 in, 2 out]
        n613 = Index Array(array=w1129, index (row)=w1135) -> (element=w1126:string[])  [unwired: 1 in]
        n614 = Index Array(array=w1126, index=0 ("索引")) -> (element=w1124:string)
        n615 = Array To Spreadsheet String(delimiter (Tab)="-" ("分隔符(Tab)"), array=w1126, 3:"" ("格式字符串")) -> ()  [unwired: 1 out]
        n616 = Get Date/Time In Seconds() -> (seconds since 1Jan1904=w1133:timestamp)
        n617 = Bundle(cluster="data in", "时间标识"=w1133, "参数"="CODMn" ("table输入"), "日志信息"=w1124, "流程参数"="" ("table输入")) -> (w1130:T2)
        n618 = call "流程日志字段定义.vi"("table输入"="操作日志", "data in"=w1130) -> ("table输出"=w1138:string, "columns"=w1139:string[], "data out"=w1140:T13)  [unwired: 7 in]
        n619 = call "插入数据.vi"("data"=w1140, "columns"=w1139, "database"="database3.mdb", "table"=w1138) -> ()  [unwired: 7 in, 1 out]
      }
    }
    n620 = Index Array(array=w953) -> (element=→"仪器时间":timestamp)  [unwired: 1 in]
    n621 = Get Date/Time In Seconds() -> (seconds since 1Jan1904=w952:timestamp)
    "系统时间" <- w952
    n622 = global read "COD读取DATA全局.vi" "data"() -> (w935:T5)
    n623 = Less Or Equal?(x=w904, y=u16 4) -> (x <= y?=w908:bool)
    n624 = global read "COD测量模式全局.vi" "测量模式"() -> (w934:string)
    n625 = Build Array(w952) -> (w951:timestamp[])
    n626 = Unbundle By Name(w935) -> ("时间"=w932:timestamp, "检测值"=w931:sgl, "数据标识"=w930:string)
    n627 = case shown="真" w908 {
      frame False {
      }
      frame True {
        n628 = local read "跨度核查标记"() -> (w1065:bool)
        n629 = local read "空白测试标记"() -> (w1064:bool)
        n630 = local read "加标回收测量"() -> (w1063:bool)
        n631 = local read "标样核查标记"() -> (w1070:bool)
        n632 = local read "零点核查标记"() -> (w1069:bool)
        n633 = local read "平行样测量"() -> (w1062:bool)
        n634 = local read "校零标记"() -> (w1061:bool)
        n635 = local read "校标标记"() -> (w1060:bool)
        n636 = local read "水样测量"() -> (w1071:bool)
        n637 = local read "测量模式数字"() -> (w1067:i32)
        n638 = Build Array(w1071, w1070, w1069, w1065, w1064, w1063, w1062, w1061, w1060) -> (w1068:bool[])
        n639 = case shown="8" w1067 {
          tunnel: ["水样测试" ("测量模式") "标样核查" ("测量模式") "零点核查" ("测量模式") "跨度核查" ("测量模式") "空白测试" ("测量模式") "加标回收" ("测量模式") "平行样" ("测量模式") "校零" ("测量模式") "校标" ("测量模式")] -> w1066
          frame 0, Default {
          }
          frame 1 {
          }
          frame 2 {
          }
          frame 3 {
          }
          frame 4 {
          }
          frame 5 {
          }
          frame 6 {
          }
          frame 7 {
          }
          frame 8 {
          }
        }
        n640 = for {
          tunnel: w1068 -> [w1082] mode=indexing
          i -> [w1081]
          n641 = case shown="真" w1082 {
            tunnel: w1081 -> [_ w1083]
            frame False {
            }
            frame True {
              "测量模式数字" <- w1083
            }
          }
        }
        n642 = global write "COD测量模式全局.vi" "测量模式"(w1066) -> ()
      }
    }
    n643 = Greater?(x=w904, y=u16 0) -> (0:w905:bool)
    n644 = call "DateToHex.vi"("DATE"=w951) -> ("数组"=w950:u16[])  [unwired: 10 in]
    n645 = call "DateToHex.vi"("DATE"=w953) -> ("数组"=w945:u16[])  [unwired: 10 in]
    n646 = call <vilib>:"Boolean Crossing PtByPt.vi"("direction"=enum16{"either", "false-true", "true-false"}."false-true", "input"=w905) -> ("crossing"=w903:bool)  [unwired: 1 in]
    n647 = local read "测量数据区"() -> (w936:T1)
    n648 = case shown="\"水样测试\"" w934 {
      tunnel: w936 -> [w1088 w1093 w1098 w1103 w1108 w1113 w1118 w1123]
      tunnel: [w1088 w1092 w1094 w1102 w1107 w1112 w1114 w1122] -> w933
      tunnel: w932 -> [_ w1091 w1097 w1101 w1106 w1111 w1117 w1121]
      tunnel: w931 -> [_ w1090 w1096 w1100 w1105 w1110 w1116 w1120]
      tunnel: w930 -> [_ w1089 w1095 w1099 w1104 w1109 w1115 w1119]
      frame "", Default {
      }
      frame "水样测试" {
        n649 = Bundle By Name(cluster=w1093, "水样数据时间"=w1091, "水样实测值"=w1090, "水样数据标识"=w1089) -> (w1092:T1)
      }
      frame "标样核查" {
        n650 = Bundle By Name(cluster=w1098, "跨度核查数据时间"=w1097, "跨度核查实测值"=w1096, "跨度核查数据标识"=w1095) -> (w1094:T1)
      }
      frame "零点核查" {
        n651 = Bundle By Name(cluster=w1103, "零点核查数据时间"=w1101, "零点核查实测值"=w1100, "零点核查数据标识"=w1099) -> (w1102:T1)
      }
      frame "加标回收" {
        n652 = Bundle By Name(cluster=w1108, "加标回收数据时间"=w1106, "加标回收实测值"=w1105, "加标回收数据标识"=w1104) -> (w1107:T1)
      }
      frame "平行样" {
        n653 = Bundle By Name(cluster=w1113, "平行样数据时间"=w1111, "平行样实测值"=w1110, "平行样数据标识"=w1109) -> (w1112:T1)
      }
      frame "校零" {
        n654 = Bundle By Name(cluster=w1118, "空白数据时间"=w1117, "空白实测值"=w1116, "空白数据标识"=w1115) -> (w1114:T1)
      }
      frame "校标" {
        n655 = Bundle By Name(cluster=w1123, "标样数据时间"=w1121, "标样实测值"=w1120, "标样数据标识"=w1119) -> (w1122:T1)
      }
    }
    "测量数据区" <- w933
    n656 = Index Array(array=w945, index=2 ("索引")) -> (element=w947:u16)
    n657 = case shown="真" w903 {
      frame False {
      }
      frame True {
        n658 = Get Date/Time In Seconds() -> (seconds since 1Jan1904=w1056:timestamp)
        "启动时间" <- w1056
        n659 = global read "COD测量模式全局.vi" "测量模式"() -> (w1057:string)
        n660 = case shown="\"加标回收\"" w1057 {
          tunnel: w1056 -> [w1058 w1059]
          frame "水样测试", Default {
            n661 = global write "COD测量模式全局.vi" "水样启动时间"(w1058) -> ()
          }
          frame "加标回收" {
            n662 = global write "COD测量模式全局.vi" "加标回收启动时间"(w1059) -> ()
          }
        }
      }
    }
    n663 = Index Array(array=w950, index=2 ("索引")) -> (element=w948:u16)
    n664 = Split Number(x=w947) -> (hi(x)=w941:u8)  [unwired: 1 out]
    n665 = call "CODMn报警信息.vi"("报警簇"=w974) -> ("CODMN报警信息"=w975:string)  [unwired: 10 in]
    n666 = Split Number(x=w948) -> (hi(x)=w944:u8)  [unwired: 1 out]
    n667 = To Byte Integer(number=w941) -> (8bit integer=w940:i8)
    n668 = To Byte Integer(number=w944) -> (8bit integer=w943:i8)
    n669 = Subtract(x=w940, y=w943) -> (x-y=w942:i8)
    n670 = feedback #2(w975) -> (w976:string)
    n671 = feedback-in #2(w975) -> ()
    n672 = Not Equal?(x=w975, y="") -> (x != y?=w980:bool)
    n673 = Absolute Value(x=w942) -> (abs(x)=w939:i8)
    n674 = Greater Or Equal?(x=w939, y=i8 5) -> (x >= y?=w937:bool)
    n675 = Not Equal?(x=w975, y=w976) -> (x != y?=w977:bool)
    n676 = case shown="真" w937 {
      tunnel: w937 -> [_ w1084]
      frame False {
      }
      frame True {
        n677 = flat-sequence {
          tunnel: w1084 -> [_]
          frame #0 {
            n678 = property on="时间校准" class="Bool (严格)"("Val(Sgnl)"=TRUE ("时间校准")) -> ()  [unwired: 2 in, 2 out]
          }
          frame #1 {
            n679 = Wait (ms)(milliseconds to wait=u32 300 ("等待时间（毫秒）")) -> ()  [unwired: 1 out]
          }
          frame #2 {
            n680 = property on="时间校准" class="Bool (严格)"("Val(Sgnl)"=FALSE ("时间校准")) -> ()  [unwired: 2 in, 2 out]
          }
        }
      }
    }
    n681 = And(x=w977, y=w980) -> (x .and. y?=w978:bool)
    n682 = case shown="真" w978 {
      tunnel: w975 -> [_ w1141]
      frame False {
      }
      frame True {
        n683 = Get Date/Time In Seconds() -> (seconds since 1Jan1904=w1143:timestamp)
        n684 = Bundle By Name(cluster=T11 {"时间标识"=timestamp(0 s since 1904-01-01), "设备"="", "日志信息"=""} ("data in"), "时间标识"=w1143, "设备"="CODMn", "日志信息"=w1141) -> (w1144:T11)
        n685 = call "报警信息字段定义.vi"("table输入"="报警信息", "data in"=w1144) -> ("table输出"=w1148:string, "columns"=w1149:string[], "data out"=w1150:T11)  [unwired: 7 in]
        n686 = call "插入数据.vi"("data"=w1150, "columns"=w1149, "database"="database3.mdb", "table"=w1148) -> ()  [unwired: 7 in, 1 out]
      }
    }
    "循环次数" <- w994
  }
  n687 = while {
    tunnel: w4 -> [w1159]
    stop <- FALSE stop-if-true
    n688 = event shown="[0] \"保存\": 鼠标按下" {
      selector: _ -> [_]
      dyn-events: _ -> [_]
      timeout: _ -> [_]
      tunnel: w1159 -> [w1169]
      event "保存": Mouse Down {
        (unwired) 1000 ("超时毫秒(-1)")
        (unwired) cluster{"starting address":u16, "values":u16[]} {"starting address"=4625, "values"=[]}
        n689 = event-data() -> ()  [unwired: 1 in, 8 out]
        n690 = local write "枚举"(enum16{"读取数据", "写入数据", "读取写入DATABASE", "读取参数"}."写入数据" ("枚举")) -> ()
        n691 = local write "水样"("水样") -> ()
        n692 = local write "标液"("标液") -> ()
        n693 = local write "硫酸"("硫酸") -> ()
        n694 = local write "恒温时间"("恒温时间") -> ()
        n695 = local write "修正系数"("修正系数") -> ()
        n696 = local write "加标回收"("加标回收") -> ()
        n697 = local write "高锰酸钾"("高锰酸钾") -> ()
        n698 = local write "基本量程"("基本量程") -> ()
        n699 = local write "标样浓度 2"("标样浓度 2") -> ()
        n700 = local write "零点泵计量数 2"("零点泵计量数 2") -> ()
        n701 = local write "标度泵计量数 2"("标度泵计量数 2") -> ()
        n702 = local write "蒸馏水"("蒸馏水") -> ()
        n703 = local write "温度 2"("温度 2") -> ()
        n704 = local write "草酸钠"("草酸钠") -> ()
        n705 = local write "质控样"("质控样") -> ()
        n706 = Build Array("温度 2", "恒温时间", "浓度", "修正系数", "基本量程", "水样", "蒸馏水", "标液", "质控样", "加标回收", "高锰酸钾", "草酸钠", "硫酸", "零点泵计量数 2", "标度泵计量数 2", "标样浓度 2") -> (w1167:dbl[])
        n707 = Bundle By Name(cluster=cluster{"starting address":u16, "values":u16[]} {"starting address"=4272, "values"=[]}, "starting address"=u16 4272, "values"=w1167) -> (w1165:cluster{"starting address":u16, "values":u16[]})
        n708 = Enqueue Element(queue=w1169, element=w1165, timeout in ms (-1)=1000 ("超时毫秒(-1)")) -> ()  [unwired: 1 in, 3 out]
      }
    }
  }
  n709 = while {
    tunnel: w8 -> [w1200]
    tunnel: w7 -> [w1199]
    tunnel: w4 -> [w1198]
    tunnel: w23 -> [w1197]
    tunnel: w22 -> [w1196]
    tunnel: [w1186] -> w21
    tunnel: [w1195] -> w20
    tunnel: w16 -> [w1193]
    tunnel: w15 -> [w1192]
    tunnel: w11 -> [w1191]
    tunnel: w10 -> [w1190]
    tunnel: w9 -> [w1189]
    tunnel: w4 -> [w1183]
    i -> [w1185]
    stop <- FALSE stop-if-true
    n710 = case shown="\"读取写入DATABASE\"" "枚举" {
      tunnel: w1200 -> [w1236 w1246 w1344 w1421]
      tunnel: w1199 -> [w1235 w1242 w1343 w1420]
      tunnel: w1198 -> [_ w1245 _ _]
      tunnel: [w1202 w1244 w1346 w1415] -> w1195
      tunnel: [w1201 w1243 w1345 w1413] -> w1186
      tunnel: w1197 -> [w1233 _ _ _]
      tunnel: w1196 -> [w1229 _ _ _]
      tunnel: w1193 -> [_ _ _ w1419]
      tunnel: w1192 -> [_ _ _ w1418]
      tunnel: w1191 -> [_ _ w1342 _]
      tunnel: w1190 -> [_ _ w1341 _]
      tunnel: w1189 -> [_ w1241 _ _]
      tunnel: w1183 -> [_ _ w1289 _]
      frame "读取数据", Default {
        n711 = Dequeue Element(queue=w1233, timeout in ms (-1)=1000 ("超时毫秒(-1)"), error in (no error)=w1229) -> (element=w1232:T6)  [unwired: 3 out]
        n712 = Unbundle By Name(w1232) -> ("starting address"=w1231:u16, "number of holding registers"=w1230:u16)
        n713 = call <vilib>:"Read Holding Registers.vi"("error in (no error)"=w1235, "quantity"=w1230, "starting address"=w1231, "MB session in"=w1236) -> ("error out"=w1224:errorcluster, "Registers"=→"Registers":u16[], "MB session out"=w1227:refnum<class "MB_Master_Serial.lvclass">)  [unwired: 5 in]
        n714 = call <vilib>:"Read Coils.vi"("error in (no error)"=w1224, "quantity"=u16 8, "starting address"=u16 140, "MB session in"=w1227) -> ("error out"=w1214:errorcluster, "Coils"=w1223:bool[], "MB session out"=w1215:refnum<class "MB_Master_Serial.lvclass">)  [unwired: 5 in]
        n715 = Index Array(array=w1223) -> (element #1=→"进水样":bool, element #2=→"进蒸馏水":bool, element #3=→"进标液":bool, element #4=→"进质控样":bool, element #5=→"进加标回收样":bool, element #6=→"进高锰酸钾":bool, element #7=→"进草酸钠":bool, element #8=→"进硫酸":bool)  [unwired: 9 in, 1 out]
        n716 = call <vilib>:"Read Coils.vi"("error in (no error)"=w1214, "quantity"=u16 1, "starting address"=u16 137, "MB session in"=w1215) -> ("error out"=w1210:errorcluster, "Coils"=w1204:bool[], "MB session out"=w1211:refnum<class "MB_Master_Serial.lvclass">)  [unwired: 5 in]
        n717 = Index Array(array=w1204) -> (element=→"搅拌":bool)  [unwired: 1 in]
        n718 = call <vilib>:"Read Coils.vi"("error in (no error)"=w1210, "quantity"=u16 1, "starting address"=u16 400, "MB session in"=w1211) -> ("error out"=w1201:errorcluster, "Coils"=w1207:bool[], "MB session out"=w1202:refnum<class "MB_Master_Serial.lvclass">)  [unwired: 5 in]
        n719 = Index Array(array=w1207) -> (element=→"加热":bool)  [unwired: 1 in]
      }
      frame "写入数据" {
        n720 = flat-sequence {
          tunnel: w1246 -> [w1257]
          tunnel: w1245 -> [w1256]
          tunnel: w1242 -> [w1250]
          tunnel: w1241 -> [w1249]
          tunnel: [w1252] -> w1240
          tunnel: [w1251] -> w1239
          tunnel: [w1248] -> w1238
          tunnel: [w1247] -> w1237
          tunnel: [w1258] -> w1243
          tunnel: [w1264] -> w1244
          tunnel: w1240 -> [w1264]
          tunnel: w1239 -> [w1258]
          tunnel: w1238 -> [w1263]
          tunnel: w1237 -> [w1262]
          frame #0 {
            n721 = Dequeue Element(queue=w1256, error in (no error)=w1249) -> (queue out=w1248:refnum<queue>, element=w1255:cluster{"starting address":u16, "values":u16[]}, error out=w1247:errorcluster)  [unwired: 1 in, 1 out]
            n722 = Unbundle By Name(w1255) -> ("starting address"=w1254:u16, "values"=w1253:u16[])
            n723 = call <vilib>:"Write Multiple Registers.vi"("error in (no error)"=w1250, "values"=w1253, "starting address"=w1254, "MB session in"=w1257) -> ("error out"=w1251:errorcluster, "MB session out"=w1252:refnum<class "MB_Master_Serial.lvclass">)  [unwired: 6 in]
          }
          frame #1 {
            n724 = Get Queue Status(queue=w1263, error in (no error)=w1262) -> (# elements in queue=w1261:i32)  [unwired: 1 in, 7 out]
            n725 = Equal To 0?(x=w1261) -> (x = 0?=w1260:bool)
            n726 = case shown="真" w1260 {
              tunnel: [enum16{"读取数据", "写入数据", "读取写入DATABASE", "读取参数"}."写入数据" ("枚举") enum16{"读取数据", "写入数据", "读取写入DATABASE", "读取参数"}."读取数据" ("枚举")] -> w1259
              tunnel: w1258 -> [_ w1266]
              frame False {
              }
              frame True {
                n727 = case shown="无错误" w1266 {
                  tunnel: ["保存成功" ("消息") "保存失败" ("消息")] -> _
                  frame No Error {
                  }
                  frame Error {
                  }
                }
              }
            }
            n728 = local write "枚举"(w1259) -> ()
          }
        }
      }
      frame "读取写入DATABASE" {
        w1311 = "CODMn" ("table")
        n729 = Dequeue Element(queue=w1342, timeout in ms (-1)=1000 ("超时毫秒(-1)"), error in (no error)=w1341) -> (element=w1349:T6)  [unwired: 3 out]
        n730 = Unbundle By Name(w1349) -> ("starting address"=w1348:u16, "number of holding registers"=w1347:u16)
        n731 = call <vilib>:"Read Holding Registers.vi"("error in (no error)"=w1343, "quantity"=w1347, "starting address"=w1348, "MB session in"=w1344) -> ("error out"=w1345:errorcluster, "Registers"=w1271:u16[], "MB session out"=w1346:refnum<class "MB_Master_Serial.lvclass">)  [unwired: 5 in]
        n732 = To Word Integer(number=w1271) -> (16bit integer=w1270:i16[])
        "DATABASE" <- w1270
        n733 = Split 1D Array(array=w1270, index=3 ("索引")) -> (first subarray=w1339:i16[], second subarray=w1328:i16[])
        n734 = global read "系统变量.vi" "运行模式"() -> (w1292:enum16{"维护模式", "常规模式", "应急模式", "质控模式"})
        n735 = case shown="\"常规模式\"" w1292 {
          tunnel: ["M" ("单位") "N" ("单位") "hd" ("单位") "hd" ("单位")] -> w1291
          frame "维护模式", Default {
          }
          frame "常规模式" {
          }
          frame "应急模式" {
          }
          frame "质控模式" {
          }
        }
        n736 = Index Array(array=w1339) -> (element #1=w1337:i16, element #2=w1336:i16, element #3=w1335:i16)  [unwired: 3 in]
        n737 = Index Array(array=w1328) -> (element #1=w1279:i16, element #2=w1332:i16, element #3=w1331:i16, element #4=w1330:i16, element #5=w1329:i16)  [unwired: 5 in]
        n738 = Index Array(array=w1328, index=6 ("索引")) -> (element=w1326:i16)
        n739 = To Single Precision Float(number=w1279) -> (single precision float=w1281:sgl)
        n740 = Divide(x=w1281, y=sgl 100.0) -> (x/y=w1280:sgl)
        n741 = Less Or Equal?(x=w1280, y=sgl 0.01) -> (x <= y?=w1284:bool)
        n742 = case shown="真" w1284 {
          tunnel: [w1404 w1405] -> w1282
          tunnel: w1280 -> [w1404 _]
          frame False {
          }
          frame True {
            n743 = Random Number (0-1)() -> (number: 0 to 1=w1408:dbl)
            n744 = Increment(x=w1408) -> (x+1=w1406:dbl)
            n745 = Divide(x=w1406, y=sgl 100.0) -> (x/y=w1405:dbl)
          }
        }
        n746 = local read "标样浓度 2"() -> (w1306:dbl)
        n747 = Build Array(w1337, w1336, w1335) -> (w1334:i16[])
        n748 = To Single Precision Float(number=w1332) -> (single precision float=w1297:sgl)
        n749 = To Single Precision Float(number=w1331) -> (single precision float=w1298:sgl)
        n750 = To Single Precision Float(number=w1330) -> (single precision float=w1299:sgl)
        n751 = To Single Precision Float(number=w1329) -> (single precision float=w1323:sgl)
        n752 = property on="基本量程" class="Enum (严格)"() -> ("Value"=w1283:enum16{"10mL", "20mL"})  [unwired: 2 in, 2 out]
        n753 = case shown="\"20mL\"" w1283 {
          tunnel: w1282 -> [w1384 w1394]
          tunnel: [w1382 w1393] -> w1272
          frame "10mL", Default {
            n754 = Less Or Equal?(x=w1384, y=2.0) -> (x <= y?=w1387:bool)
            n755 = Greater?(x=w1384, y=0.0) -> (0:w1386:bool)
            n756 = And(x=w1387, y=w1386) -> (x .and. y?=w1383:bool)
            n757 = case shown="真" w1383 {
              tunnel: w1384 -> [w1389 w1392]
              tunnel: [w1389 w1390] -> w1382
              frame False {
              }
              frame True {
                n758 = Multiply(x=w1392, y=1.1) -> (x*y=w1390:dbl)
              }
            }
          }
          frame "20mL" {
            n759 = Greater?(x=w1394, y=0.0) -> (0:w1397:bool)
            n760 = Less Or Equal?(x=w1394, y=5.0) -> (x <= y?=w1398:bool)
            n761 = And(x=w1398, y=w1397) -> (x .and. y?=w1395:bool)
            n762 = case shown="假" w1395 {
              tunnel: w1394 -> [w1400 w1403]
              tunnel: [w1400 w1401] -> w1393
              frame False {
              }
              frame True {
                n763 = Multiply(x=w1403, y=1.2) -> (x*y=w1401:dbl)
              }
            }
          }
        }
        "COD浓度（mg/L)" <- w1272
        n764 = Divide(x=w1306, y=100.0) -> (x/y=w1296:dbl)
        n765 = To Single Precision Float(number=w1326) -> (single precision float=w1286:sgl)
        n766 = call "HexToDate.vi"("数组"=w1334) -> ("DATE"=w1338:timestamp[])  [unwired: 10 in]
        n767 = global read "COD测量模式全局.vi" "测量模式"() -> (w1287:string)
        n768 = global read "COD测量模式全局.vi" "测量模式"() -> (w1278:string)
        n769 = Divide(x=w1323, y=sgl 1000.0) -> (x/y=w1300:sgl)
        n770 = Index Array(array=w1338) -> (element=w1333:timestamp)  [unwired: 1 in]
        n771 = Format Into String(format string="w%05d" ("格式字符串"), u32 1019 ("因子编码")) -> (resulting string=w1295:string)  [unwired: 2 in, 1 out]
        n772 = Not Equal?(x=w1278, y="校标") -> (x != y?=w1276:bool)
        n773 = case shown="真" w1276 {
          tunnel: w1289 -> [_ w1363]
          tunnel: w1272 -> [_ w1361]
          frame False {
            n774 = local write "枚举"(enum16{"读取数据", "写入数据", "读取写入DATABASE", "读取参数"}."读取数据" ("枚举")) -> ()
          }
          frame True {
            n775 = Greater Or Equal?(x=w1361, y=10.0) -> (x >= y?=w1359:bool)
            n776 = case shown="真" "自动切换量程" {
              tunnel: w1363 -> [_ w1366]
              tunnel: w1359 -> [_ w1365]
              frame False {
                n777 = local write "枚举"(enum16{"读取数据", "写入数据", "读取写入DATABASE", "读取参数"}."读取数据" ("枚举")) -> ()
              }
              frame True {
                n778 = case shown="真" w1365 {
                  tunnel: w1366 -> [w1368 w1376]
                  frame False {
                    # "自动切换量程"
                    n779 = local write "枚举"(enum16{"读取数据", "写入数据", "读取写入DATABASE", "读取参数"}."写入数据" ("枚举")) -> ()
                    n780 = Bundle By Name(cluster=cluster{"starting address":u16, "values":u16[]} {"starting address"=0, "values"=[]}, "starting address"=u16 4276, "values"=u16[] [0]) -> (w1371:cluster{"starting address":u16, "values":u16[]})
                    n781 = Enqueue Element(queue=w1368, element=w1371) -> ()  [unwired: 2 in, 3 out]
                  }
                  frame True {
                    n782 = local write "枚举"(enum16{"读取数据", "写入数据", "读取写入DATABASE", "读取参数"}."写入数据" ("枚举")) -> ()
                    n783 = Bundle By Name(cluster=cluster{"starting address":u16, "values":u16[]} {"starting address"=0, "values"=[]}, "starting address"=u16 4276, "values"=u16[] [1]) -> (w1377:cluster{"starting address":u16, "values":u16[]})
                    n784 = Enqueue Element(queue=w1376, element=w1377) -> ()  [unwired: 2 in, 3 out]
                  }
                }
              }
            }
          }
        }
        n785 = local read "温度"() -> (w1290:dbl)
        n786 = global read "COD测量模式全局.vi" "测量模式"() -> (w1275:string)
        n787 = Bundle(cluster=T5 {"时间"=timestamp(0 s since 1904-01-01), "测量模式"="", "数据类型"="", "检测值"=0.0, "单位"="", "数据标识"="", "因子编码"="", "标样参考值"=0.0, "ORP-A"=0.0, "ORP-B"=0.0, "ORP-K"=0.0, "COD滴定值"=0.0, "高锰酸钾滴定数"=0.0, "温度"=0.0} ("data"), "时间"=w1333, "测量模式"=w1287, "数据类型"=w1291, "检测值"=w1272, "单位"="mg/L", "数据标识"="N", "因子编码"=w1295, "标样参考值"=w1296, "ORP-A"=w1297, "ORP-B"=w1298, "ORP-K"=w1299, "COD滴定值"=w1300, "高锰酸钾滴定数"=w1286, "温度"=w1290) -> (w1288:T5)
        "data" <- w1288
        n788 = Build Array("时间", "测量模式", "数据类型", "检测值", "单位", "数据标识", "因子编码", "标样参考值", "ORPA", "ORPB", "ORPK", "COD滴定值", "高锰酸钾滴定数", "温度") -> (w1310:string[])
        "columns" <- w1310
        n789 = Equal?(x=w1275, y="校标") -> (x = y?=w1273:bool)
        n790 = global write "COD浓度全局变量.vi" "COD浓度（mg/L)"(w1272) -> ()
        n791 = global write "COD读取DATA全局.vi" "data"(w1288) -> ()
        n792 = flat-sequence {
          tunnel: w1311 -> [w1381]
          tunnel: w1310 -> [w1380]
          tunnel: w1288 -> [w1379]
          frame #0 {
            n793 = call "数据写入database.vi"("data"=w1379, "columns"=w1380, "table"=w1381) -> ()  [unwired: 8 in, 1 out]
          }
        }
        n794 = case shown="真" w1273 {
          tunnel: w1286 -> [_ w1350]
          frame False {
          }
          frame True {
            n795 = local read "当前校准"() -> (w1351:i32)
            n796 = case shown="1, 默认" w1351 {
              tunnel: w1350 -> [w1352 w1353 w1354 w1355 w1356 w1357]
              frame 1, Default {
                n797 = local write "泵滴定数1"(w1352) -> ()
              }
              frame 2 {
                n798 = local write "泵滴定数2"(w1353) -> ()
              }
              frame 3 {
                n799 = local write "泵滴定数3"(w1354) -> ()
              }
              frame 4 {
                n800 = local write "泵滴定数4"(w1355) -> ()
              }
              frame 5 {
                n801 = local write "泵滴定数5"(w1356) -> ()
              }
              frame 6 {
                n802 = local write "泵滴定数6"(w1357) -> ()
              }
            }
          }
        }
        "table 输入" <- w1311
      }
      frame "读取参数" {
        n803 = Dequeue Element(queue=w1419, timeout in ms (-1)=1000 ("超时毫秒(-1)"), error in (no error)=w1418) -> (element=w1425:T6)  [unwired: 3 out]
        n804 = local write "枚举"(enum16{"读取数据", "写入数据", "读取写入DATABASE", "读取参数"}."读取数据" ("枚举")) -> ()
        n805 = Unbundle By Name(w1425) -> ("starting address"=w1424:u16, "number of holding registers"=w1423:u16)
        n806 = local read "读取KB值"() -> (w1414:bool)
        n807 = call <vilib>:"Read Holding Registers.vi"("error in (no error)"=w1420, "quantity"=w1423, "starting address"=w1424, "MB session in"=w1421) -> ("error out"=w1413:errorcluster, "Registers"=w1417:u16[], "MB session out"=w1415:refnum<class "MB_Master_Serial.lvclass">)  [unwired: 5 in]
        "读取参数" <- w1417
        n808 = case shown="真" w1414 {
          tunnel: w1417 -> [w1435 w1460]
          tunnel: w1413 -> [_ w1462]
          frame False {
            n809 = Index Array(array=w1435) -> (element #1=w1429:u16, element #2=w1448:u16, element #3=w1447:u16, element #4=w1427:u16, element #5=w1446:u16, element #6=w1445:u16, element #7=w1444:u16, element #8=w1443:u16, element #9=w1442:u16, element #10=w1441:u16, element #11=w1440:u16, element #12=w1439:u16, element #13=w1438:u16, element #14=w1437:u16, element #15=w1436:u16, element #16=w1434:u16)  [unwired: 16 in]
            n810 = local write "浓度"(w1447) -> ()
            n811 = local write "水样"(w1445) -> ()
            n812 = local write "硫酸"(w1438) -> ()
            n813 = local write "标液"(w1443) -> ()
            n814 = Divide(x=w1429, y=u16 10) -> (x/y=w1430:dbl)
            n815 = local write "草酸钠"(w1439) -> ()
            n816 = local write "蒸馏水"(w1444) -> ()
            n817 = local write "质控样"(w1442) -> ()
            n818 = local write "恒温时间"(w1448) -> ()
            n819 = local write "基本量程"(w1446) -> ()
            n820 = local write "加标回收"(w1441) -> ()
            n821 = local write "高锰酸钾"(w1440) -> ()
            n822 = local write "零点泵计量数 2"(w1437) -> ()
            n823 = local write "标度泵计量数 2"(w1436) -> ()
            n824 = Divide(x=w1427, y=u16 100) -> (x/y=w1426:dbl)
            n825 = Divide(x=w1434, y=u16 100) -> (x/y=w1433:dbl)
            n826 = local write "温度"(w1430) -> ()
            n827 = local write "修正系数 2"(w1426) -> ()
            n828 = local write "浓度 2"(w1433) -> ()
          }
          frame True {
            (unwired) 9 ("索引")
            n829 = case shown="错误" w1462 {
              tunnel: ["读取成功" ("消息") "读取失败" ("消息")] -> w1461
              frame No Error {
              }
              frame Error {
              }
            }
            n830 = Array Subset(array=w1460, index=10 ("索引"), length=12 ("长度")) -> (w1457:u16[])
            n831 = call "浮点CDAB转换COD.vi"("数组"=w1457) -> ("数组 2"=w1456:sgl[])  [unwired: 10 in]
            n832 = One Button Dialog(message=w1461) -> ()  [unwired: 1 in, 1 out]
            n833 = Array To Cluster(array=w1456) -> (cluster=w1455:T14)
            n834 = local read "量程选择"() -> (w1449:enum16{"低量程", "高量程"})
            n835 = case shown="\"高量程\"" w1449 {
              tunnel: w1455 -> [w1466 w1470]
              tunnel: [w1465 w1469] -> w1452
              tunnel: [w1464 w1468] -> w1451
              tunnel: [w1463 w1467] -> w1450
              frame "低量程", Default {
                n836 = Unbundle By Name(w1466) -> ("数组 2[2]"=w1465:sgl, "数组 2[0]"=w1464:sgl, "数组 2[1]"=w1463:sgl)
              }
              frame "高量程" {
                n837 = Unbundle By Name(w1470) -> ("数组 2[5]"=w1469:sgl, "数组 2[3]"=w1468:sgl, "数组 2[4]"=w1467:sgl)
              }
            }
            n838 = Bundle By Name(cluster=cluster{"X^2":dbl, "X":dbl, "b":dbl} {"X^2"=0.0, "X"=0.0, "b"=0.0} ("方程系数"), "X^2"=w1452, "X"=w1451, "b"=w1450) -> (w1453:cluster{"X^2":dbl, "X":dbl, "b":dbl})
            n839 = local write "方程系数"(w1453) -> ()
          }
        }
      }
    }
    n840 = Unbundle By Name(w1186) -> ("status"=w1187:bool)
    n841 = Not(x=w1187) -> (.not. x?=→"通讯状态":bool)
    "数值" <- w1185
  }
  n842 = call-dynamic "Close Session.vi"("error in (no error)"=w21, "MB_Serial session"=w20) -> ()  [unwired: 9 in, 1 out]
